vi "main 0.9.2.vi"() -> ()   [LabVIEW 2020]
uses:
  subvi/Newport ESP301/Newport ESP301.lvlib
  subvi/sp_manip.llb/sp_manip_lib.lvlib
  subvi/sp_manip.llb/tcp_gateway.lvlib
  subvi/PHOIBOS/DEFINITIONS/DEF_dev_type.ctl
  subvi/PHOIBOS/DEFINITIONS/DEF_dev_state.ctl
  <vilib>/Utility/file.llb/Write Delimited Spreadsheet (DBL).vi
  <vilib>/Utility/file.llb/Read Delimited Spreadsheet (string).vi
  <vilib>/Analysis/NI_AALBase.lvlib
  <vilib>/Analysis/1siggen.llb/Ramp Pattern by Samples.vi
  <vilib>/DAQmx/create/channels.llb/DAQmx Create Channel (AI-Voltage-Basic).vi
panel:
  in  "Frame trigger \n(High Performance and QE only)":u16
  in  "Operating mode\nHP & QE / HS & DiCam Pro":u32=1
  out "Waveform Chart":dbl(graph)=205.72
  out "G2 X":cluster{dbl[], "Ramp Pattern":dbl[]}(graph)
  in  "reset every n pics":bool=TRUE
  in  "pics2avg":i32=20
  in  "abort acq.":bool
  out "G2 Y":cluster{dbl[], "Ramp Pattern":dbl[]}(graph)={[0.0, 0.0, 0.0, 0.0, 0.0, 0.0, 0.0, 0.0, 0.0, 0.0, 0.0, 0.0, 0.0, 0.0, 0.0, 0.0, 0.0, 0.0, 0.0, 0.0, 0.0, 0.0, 0.0, 0.0, 0.0, 0.0, 0.0, 0.0, 0.0, 0.0, 0.0, 0.0, 0.0, 0.0, 0.0, 0.0, 0.0, 0.0, 0.0, 0.0, 0.0, 0.0, 0.0, 0.0, 0.0, 0.0, 0.0, 0.0, 0.0, 0.0, 0.0, 0.0, 0.0, 0.0, 0.0, 0.0, 0.0, 0.0, 0.0, 0.0, 0.0, 0.0, 0.0, 0.0, 0.0, 0.0, 0.0, 0.0, 0.0, 0.0, 0.0, 0.0, 0.0, 0.0, 0.0, 0.0, 0.0, 28.048333333333332, 101.45500000000001, 63.635000000000005, 12.581666666666669, 0.0, 0.0, 0.0, 0.0, 0.0, 0.0, 0.0, 0.0, 0.0, 0.0, 0.0, 0.0, 0.0, 0.0, 0.0, 0.0, 0.0, 0.0, 0.0, 0.0, 0.0, 0.0, 0.0, 0.0, 0.0, 0.0, 0.0, 0.0, 0.0, 0.0, 0.0, 0.0, 0.0, 0.0, 0.0, 0.0, 0.0, 0.0, 0.0, 0.0, 0.0, 0.0, 0.0, 0.0, 0.0, 0.0, 0.0, 0.0, 0.0, 0.0, 0.0, 0.0, 0.0, 0.0, 0.0, 0.0, 0.0, 0.0, 0.0, 0.0, 0.0, 0.0, 0.0, 0.0, 0.0, 0.0, 0.0, 0.0, 0.0, 0.0, 0.0, 0.0, 0.0, 0.0, 0.0, 0.0, 0.0, 0.0, 0.0, 0.0, 0.0, 0.0, 0.0, 0.0, 0.0, 0.0, 0.0, 0.0, 0.0, 0.0, 0.0, 0.0, 0.0, 0.0, 0.0, 0.0, 0.0, 0.0, 0.0, 0.0, 0.0, 0.0, 0.0, 0.0, 0.0, 0.0, 0.0, 0.0, 0.0, 0.0, 0.0, 0.0, 0.0, 0.0, 0.0, 0.0, 0.0, 0.0, 0.0, 0.0, 0.0, 0.0, 0.0, 0.0, 0.0, 0.0, 0.0, 0.0, 0.0, 0.0, 0.0, 0.0, 0.0, 0.0, 0.0, 0.0, 0.0, 0.0, 0.0, 0.0, 0.0, 0.0, 0.0, 0.0, 0.0, 0.0, 0.0, 0.0, 0.0, 0.0, 0.0, 0.0, 0.0, 0.0, 0.0, 0.0, 0.0, 0.0, 0.0, 0.0, 0.0, 0.0, 0.0, 0.0, 0.0, 0.0, 0.0, 0.0, 0.0, 0.0, 0.0, 0.0, 0.0, 0.0, 0.0], "Ramp Pattern"=[0.0, 1.003921568627451, 2.007843137254902, 3.011764705882353, 4.015686274509804, 5.019607843137255, 6.023529411764706, 7.027450980392157, 8.031372549019608, 9.035294117647059, 10.03921568627451, 11.04313725490196, 12.047058823529412, 13.050980392156863, 14.054901960784314, 15.058823529411764, 16.062745098039215, 17.066666666666666, 18.070588235294117, 19.07450980392157, 20.07843137254902, 21.08235294117647, 22.08627450980392, 23.090196078431372, 24.094117647058823, 25.098039215686274, 26.101960784313725, 27.105882352941176, 28.109803921568627, 29.113725490196078, 30.11764705882353, 31.12156862745098, 32.12549019607843, 33.129411764705885, 34.13333333333333, 35.13725490196079, 36.141176470588235, 37.14509803921569, 38.14901960784314, 39.15294117647059, 40.15686274509804, 41.16078431372549, 42.16470588235294, 43.168627450980395, 44.17254901960784, 45.1764705882353, 46.180392156862744, 47.1843137254902, 48.188235294117646, 49.1921568627451, 50.19607843137255, 51.2, 52.20392156862745, 53.207843137254905, 54.21176470588235, 55.21568627450981, 56.219607843137254, 57.22352941176471, 58.227450980392156, 59.23137254901961, 60.23529411764706, 61.23921568627451, 62.24313725490196, 63.247058823529414, 64.25098039215686, 65.25490196078431, 66.25882352941177, 67.26274509803922, 68.26666666666667, 69.27058823529411, 70.27450980392157, 71.27843137254902, 72.28235294117647, 73.28627450980392, 74.29019607843138, 75.29411764705883, 76.29803921568627, 77.30196078431372, 78.30588235294118, 79.30980392156863, 80.31372549019608, 81.31764705882352, 82.32156862745099, 83.32549019607843, 84.32941176470588, 85.33333333333333, 86.33725490196079, 87.34117647058824, 88.34509803921569, 89.34901960784313, 90.3529411764706, 91.35686274509804, 92.36078431372549, 93.36470588235294, 94.3686274509804, 95.37254901960785, 96.37647058823529, 97.38039215686274, 98.3843137254902, 99.38823529411765, 100.3921568627451, 101.39607843137254, 102.4, 103.40392156862745, 104.4078431372549, 105.41176470588235, 106.41568627450981, 107.41960784313726, 108.4235294117647, 109.42745098039215, 110.43137254901961, 111.43529411764706, 112.43921568627451, 113.44313725490196, 114.44705882352942, 115.45098039215686, 116.45490196078431, 117.45882352941176, 118.46274509803922, 119.46666666666667, 120.47058823529412, 121.47450980392156, 122.47843137254903, 123.48235294117647, 124.48627450980392, 125.49019607843137, 126.49411764705883, 127.49803921568628, 128.50196078431372, 129.50588235294117, 130.50980392156862, 131.51372549019607, 132.51764705882354, 133.521568627451, 134.52549019607844, 135.52941176470588, 136.53333333333333, 137.53725490196078, 138.54117647058823, 139.54509803921567, 140.54901960784315, 141.5529411764706, 142.55686274509804, 143.5607843137255, 144.56470588235294, 145.5686274509804, 146.57254901960783, 147.57647058823528, 148.58039215686276, 149.5843137254902, 150.58823529411765, 151.5921568627451, 152.59607843137255, 153.6, 154.60392156862744, 155.6078431372549, 156.61176470588236, 157.6156862745098, 158.61960784313726, 159.6235294117647, 160.62745098039215, 161.6313725490196, 162.63529411764705, 163.6392156862745, 164.64313725490197, 165.64705882352942, 166.65098039215687, 167.65490196078431, 168.65882352941176, 169.6627450980392, 170.66666666666666, 171.6705882352941, 172.67450980392158, 173.67843137254903, 174.68235294117648, 175.68627450980392, 176.69019607843137, 177.69411764705882, 178.69803921568626, 179.7019607843137, 180.7058823529412, 181.70980392156864, 182.71372549019608, 183.71764705882353, 184.72156862745098, 185.72549019607843, 186.72941176470587, 187.73333333333332, 188.7372549019608, 189.74117647058824, 190.7450980392157, 191.74901960784314, 192.75294117647059, 193.75686274509803, 194.76078431372548, 195.76470588235293, 196.7686274509804, 197.77254901960785, 198.7764705882353, 199.78039215686275, 200.7843137254902, 201.78823529411764, 202.7921568627451, 203.79607843137254, 204.8, 205.80392156862746, 206.8078431372549, 207.81176470588235, 208.8156862745098, 209.81960784313725, 210.8235294117647, 211.82745098039214, 212.83137254901962, 213.83529411764707, 214.8392156862745, 215.84313725490196, 216.8470588235294, 217.85098039215686, 218.8549019607843, 219.85882352941175, 220.86274509803923, 221.86666666666667, 222.87058823529412, 223.87450980392157, 224.87843137254902, 225.88235294117646, 226.8862745098039, 227.89019607843136, 228.89411764705883, 229.89803921568628, 230.90196078431373, 231.90588235294118, 232.90980392156862, 233.91372549019607, 234.91764705882352, 235.92156862745097, 236.92549019607844, 237.9294117647059, 238.93333333333334, 239.93725490196078, 240.94117647058823, 241.94509803921568, 242.94901960784313, 243.95294117647057, 244.95686274509805, 245.9607843137255, 246.96470588235294, 247.9686274509804, 248.97254901960784, 249.9764705882353, 250.98039215686273, 251.98431372549018, 252.98823529411766, 253.9921568627451, 254.99607843137255, 256.0]}
  out "ETA":timestamp=timestamp(3548431207.455768 s since 1904-01-01) format="%<%H:%M:%S>T"
  out "acq. imgs":i32=50
  out "snap_prog":dbl(slide)=1.0 scale=0.0..1.0
  in  "BasePath":path=path "Z:/PESdata"
  in  "cam_liveavg":bool=TRUE caption="live average"
  out "cam_fps":dbl=19.76375300099574 caption="FPS" format="%.1g"
  out "sideimg":dbl[][](graph)
  in  "RunNumber":u16=145
  out "sum":dbl=205.72 format="%#.2g"
  out "max":dbl=120.33666666666666
  out "mainimg":dbl[][](graph)
  out "ESP_con?":bool=TRUE caption="ESP301"
  out "phoib_con?":bool caption="PHOIBOS"
  out "manip_con?":bool caption="manipulator"
  out "cam_con?":bool caption="camera"
  in  "main_close":bool
  in  "Tab Control":T1(tab)
  in  "manip_deltas":dbl[](array[numeric])=[0.0, 0.0, 0.0, 0.0, 10.0, 0.0] caption="delta" format="%#.5g"
  in  "aq.mode":enum32{"Radio Selection 1", "Radio Selection 2"}(radio)=enum."Radio Selection 2"
  in  "dark avg":i32=100
  in  "averages":i32=50 caption="N"
  in  "ESP_delta":dbl=0.0015 caption="relative [mm]"
  in  "ESP_-":bool
  in  "ESP_+":bool
  in  "ESP_go":bool
  in  "ESP_dest_t":dbl=-1000.0 caption="[fs]"
  in  "ESP_dest":dbl=26.730803771 caption="[mm]"
  in  "ESP_set_t0":bool
  in  "phoib_I_6s":dbl=3200.0
  in  "phoib_I_5s":dbl=1500.0
  in  "phoib_I_4s":dbl=4.558
  in  "phoib_I_3s":dbl=-7.0
  in  "phoib_I_2s":dbl=20.0
  in  "phoib_I_1s":dbl=22.0
  in  "phoib_standby":bool
  in  "phoib_set":bool
  out "phoib_I_6":dbl=3200.0 caption="Screen Voltage"
  out "phoib_I_5":dbl=1500.0 caption="Detctor Voltage"
  out "phoib_I_4":dbl=4.558 caption="Work Function"
  out "phoib_I_3":dbl=-7.0 caption="Coil Current"
  out "phoib_I_2":dbl=20.0 caption="Pass Energy"
  out "phoib_I_1":dbl=22.0 caption="Kinetic Energy"
  out "Saved Positions":string[][](table)=[["ertwertwert", "-2.299945", "-2.030214", "38.900024", "50.000762", "0.000887", "-97.998082"], ["uztgugt", "-14.999451", "-13.638894", "442.380066", "13.998380", "-1.893758", "-76.305838"], ["asdf", "-14.999451", "-13.638894", "442.380066", "13.998380", "-1.893758", "-76.305838"], ["test3", "-14.999451", "-13.638894", "441.380066", "13.998380", "-1.893758", "-76.305838"]]
  in  "Save Pos":bool
  in  "Load":bool
  in  "Delete":bool
  in  "ManipRel +":bool
  in  "ManipRel -":bool
  in  "Move Abs":bool
  in  "stop manip":bool
  in  "dest":dbl[](array[numeric])=[-2.6172862113166087, -0.009888298846365134, 68.5008544921875, -46.36280498847848, 1.1073518432055398, -218.56360350415366] caption="destination" format="%#.5g"
  out "axis":string[](array[string])=["x", "y", "z", "polar", "tilt", "azimut"]
  out "pos":dbl[](array[numeric]) caption="position" format="%.5f"
  in  "Mode":T2(ring)=enum."WideAngleMode"
  in  "VoltageRange":enum16{"3.5kV", "1.5kV", "400V", "100V", "10V"}(ring)=enum."400V"
  out "ESP_pos":dbl=26.86195 caption="Position"
  out "ESP_delay":dbl=-125.08653569931175 caption="Delay"
  out "ESP_t0":dbl=26.8807 caption="Time Zero @"
  out "phoib_I_7":dbl=-17.0 caption="Conversion Voltage"
  in  "phoib_I_7s":dbl=-17.0
  in  "phoib_I_8s":dbl=0.0039
  in  "phoib_I_9s":dbl=0.0039
  out "phoib_I_8":dbl=0.0039 caption="FD1"
  out "phoib_I_9":dbl=0.0039 caption="FD2"
  in  "gain":bool
  in  "exposure [ms]":u32=50
  in  "binning":u16(ring)=2 items=["X 1", "X 2", "X 4", "X 8"]
  in  "cam_dark?":bool=TRUE caption="subtract dark?"
  in  "cam_dark":bool
  in  "cam_saveimg":bool
  in  "e-size":u8
  in  "lower threshold":i32=50
  in  "count?":bool
  in  "ROI Left":i32=1
  in  "ROI Right":i32=43
  in  "ROI Top":i32=1
  in  "ROI Bottom":i32=33
  out "moving?":bool[](array[boolean])
  out "del_ETA":timestamp=timestamp(3548447168.6093655 s since 1904-01-01) format="%<%H:%M:%S>T"
  out "time / step":dbl=3.7475930503989816
  out "duration [HH:MM:SS]":dbl=47385.71071624756 format="%<%H:%M:%S>t"
  out "disk [MB]":dbl=5419.953
  out "RAM [MB]":dbl=27.097
  out "total steps":dbl=9800.0
  out "delaypoints":dbl=49.0
  in  "generate delay table":bool
  in  "load delay table":bool
  in  "delay table [fs]":string[][](table)=[["-200.000000"], ["-175.000000"], ["-150.000000"], ["-125.000000"], ["-100.000000"], ["-75.000000"], ["-50.000000"], ["-25.000000"], ["0.000000"], ["25.000000"], ["50.000000"], ["75.000000"], ["100.000000"], ["125.000000"], ["150.000000"], ["175.000000"], ["200.000000"], ["225.000000"], ["250.000000"], ["275.000000"], ["300.000000"], ["325.000000"], ["350.000000"], ["375.000000"], ["400.000000"], ["425.000000"], ["450.000000"], ["475.000000"], ["500.000000"], ["525.000000"], ["550.000000"], ["575.000000"], ["600.000000"], ["625.000000"], ["650.000000"], ["675.000000"], ["700.000000"], ["725.000000"], ["750.000000"], ["775.000000"], ["800.000000"], ["825.000000"], ["850.000000"], ["875.000000"], ["900.000000"], ["925.000000"], ["950.000000"], ["975.000000"], ["1000.000000"]]
  in  "delscan_iters":u32=200 caption="iterations"
  out "scangraph":cluster{"delaypoints":dbl[], dbl[]}(graph)={"delaypoints"=[-200.0, -175.0, -150.0, -125.0, -100.0, -75.0, -50.0, -25.0, 0.0, 25.0, 50.0, 75.0, 100.0, 125.0, 150.0, 175.0, 200.0, 225.0, 250.0, 275.0, 300.0, 325.0, 350.0, 375.0, 400.0, 425.0, 450.0, 475.0, 500.0, 525.0, 550.0, 575.0, 600.0, 625.0, 650.0, 675.0, 700.0, 725.0, 750.0, 775.0, 800.0, 825.0, 850.0, 875.0, 900.0, 925.0, 950.0, 975.0, 1000.0], [21425.231929824553, 20846.290614035148, 20035.560438596513, 18931.235614035082, 19640.659557522133, 21305.676814159116, 29251.80778761067, 69089.9434513275, 126421.4030973446, 163646.65610619384, 171927.22929203612, 157521.9204424778, 146716.11486725596, 135894.3418584061, 130437.91398230121, 119156.57761061934, 115502.62300884936, 103421.47973451365, 100060.49123893768, 93085.71787610617, 90135.85805309749, 86817.93584070833, 80391.69256637139, 77159.11646017693, 77729.56053097341, 73257.13840707966, 70575.97486725691, 66315.25460177004, 66705.37823008854, 63696.19292035409, 61819.46247787618, 60200.33123893791, 57469.7140707966, 55306.85336283208, 53731.13327433622, 50220.71699115046, 51078.037433628335, 47817.420265486544, 47812.83389380534, 46146.23106194685, 44534.275398229904, 42332.0369026551, 45537.85681415925, 40834.3, 41967.50035398256, 40596.04380530956, 39278.89221238937, 39217.73823008859, 37653.17115044236]}
  in  "delscan_abort":bool
  out "delscan_progress":u32(slide)=4 scale=0.0..49.0
  in  "delscan_go":bool
  out "delscan_pos":dbl=26.861962971375 caption="stage pos [mm]"
  in  "delscan_end":dbl=1000.0 caption="end [fs]"
  in  "delscan_stepsize":dbl=25.0 caption="stepsize [fs]"
  in  "delscan_start":dbl=-200.0 caption="start [fs]"
  out "iteration":i32=114
  in  "delscan_finishIteration":bool
  in  "manip_scan_steps":u32=3
  in  "Optimize":bool
  in  "manip_scan_delta":dbl[](array[numeric])=[0.0, 0.0, 0.0, 0.0, 1.0, 0.0] caption="delta" format="%#.5g"
  out "delscan_progress 2":u32(slide)=2 scale=0.0..3.0
  in  "abort":bool
  in  "dev_bench":bool
  out "x/y":dbl
  out "1/x":dbl
  in  "stop":bool
  out "voltage out":dbl
  out "sideimg 2":i32[][](graph)
  in  "manip_init":bool
  in  "manip_release":bool
  in  "phoib_init":bool
  in  "phoib_release":bool
  in  "ESP_init":bool
  in  "ESP_release":bool
  in  "ESP301 VISA":refnum<visa-resource-name>="COM8"
  in  "board number":i32
  in  "cam_init":bool
  in  "cam_release":bool
  out "cam_error":errorcluster
  out "phoib_error":errorcluster
  out "state":T3=1 items=["Off"=-1, "Standby"=0, "On"=1]
  in  "ESP Axis":i32=1 min=1 max=3
  out "error out":errorcluster
  out "error out 2":errorcluster={"status"=TRUE, "code"=1, "source"="TCP Write in sp_manip_lib.lvlib:sp_manip_disconnect.vi->main 0.9.2.vi"}
  # "0 = sequential\n1 = simultaneous"
  # "0 = internal\n1 = external rising\n2 = external falling"
  # "camera"
  # "analyzer"
  # "manipulator"
  # "aquisition"
  # "delay stage"
  # "Position"
  # "Destination"
  # "X\nY\nZ\npolar\ntilt\nazimut"
  # "camera"
  # "phoibos"
  # "ESP301"
  # "manipulator"
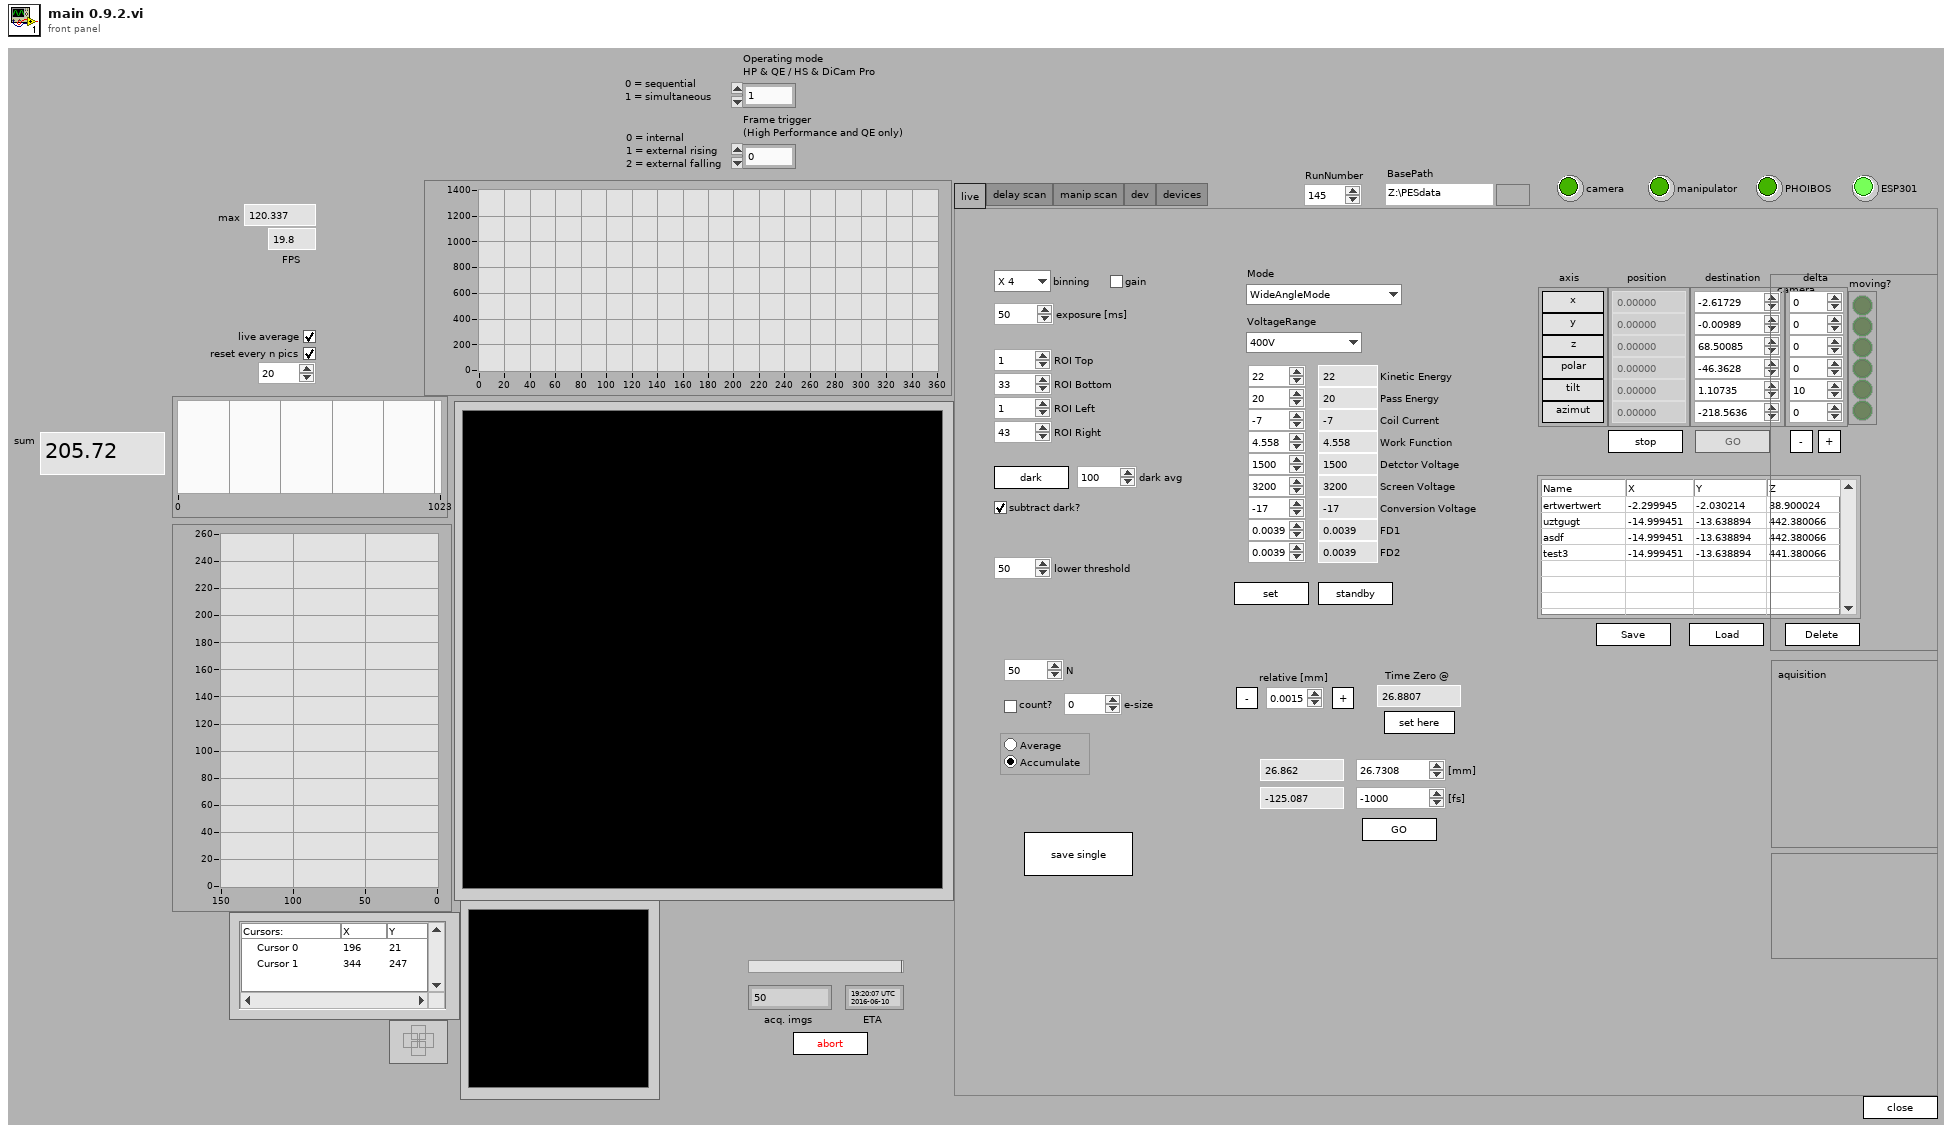
[diagram p1: front panel]
types:
  T1 = enum32{"live", "delay scan", "manip scan", "dev", "devices"}
  T2 = enum16{"HighMagnification", "MediumMagnification", "LowMagnification", "HighAngularDispersion", "MediumAngularDispersion", "LowAngularDispersion", "WideAngleMode", "LargeArea", "MediumArea", "SmallArea", "HighMagnification2", "SmallArea2", "ImagingMode"}
  T3 = typedef "DEF_dev_state.ctl" = i32
  T4 = typedef "LVCursorListTypeDef.ctl" = cluster{"Name":string, "Color":u32, "Style":u8, "Point Style":u8, "Name Visible":bool, "Allow Drag":bool, "Cursor Mode":u32, "Plot":i32, "Index":i32, "Position":cluster{"X":dbl, "Y":dbl}, "X Scale":u32, "Y Scale":u32, "Watch Plots":i32[], "Watch All Plots":bool, "Plot Area":i32, "Label Offset":cluster{"X":dbl, "Y":dbl}}[]
  T5 = cluster{"delay pointss [fs]":dbl[], "Intensity Chart":dbl[]}
  T6 = cluster{"Camera type":u32, "Operating mode\nHP & QE / HS & DiCam Pro ":u32, "Frame trigger \n(High Performance and QE only)":u16, "Sequence trigger":u16, "Low Light\n(QE only)":bool, "Gain":bool, "Horzontal\nbinning":u16, "Vertical\nbinning ":u16, "ROI Left":i32, "ROI Right":i32, "ROI Top":i32, "ROI Bottom":i32}
  T7 = cluster{"Name":string, "Color":u32, "Style":u8, "Point Style":u8, "Name Visible":bool, "Allow Drag":bool, "Cursor Mode":u32, "Plot":i32, "Index":i32, "Position":cluster{"X":dbl, "Y":dbl}, "X Scale":u32, "Y Scale":u32, "Watch Plots":i32[], "Watch All Plots":bool, "Plot Area":i32, "Label Offset":cluster{"X":dbl, "Y":dbl}}
  T8 = cluster{"Axis_Name":string, "Axis_Type":string, "Axis_Position":dbl, "continous":bool, "moving":bool}[]
  T9 = typedef "DEF_dev_type.ctl" = enum32{"devA (analyzer)", "devD (detector)"}
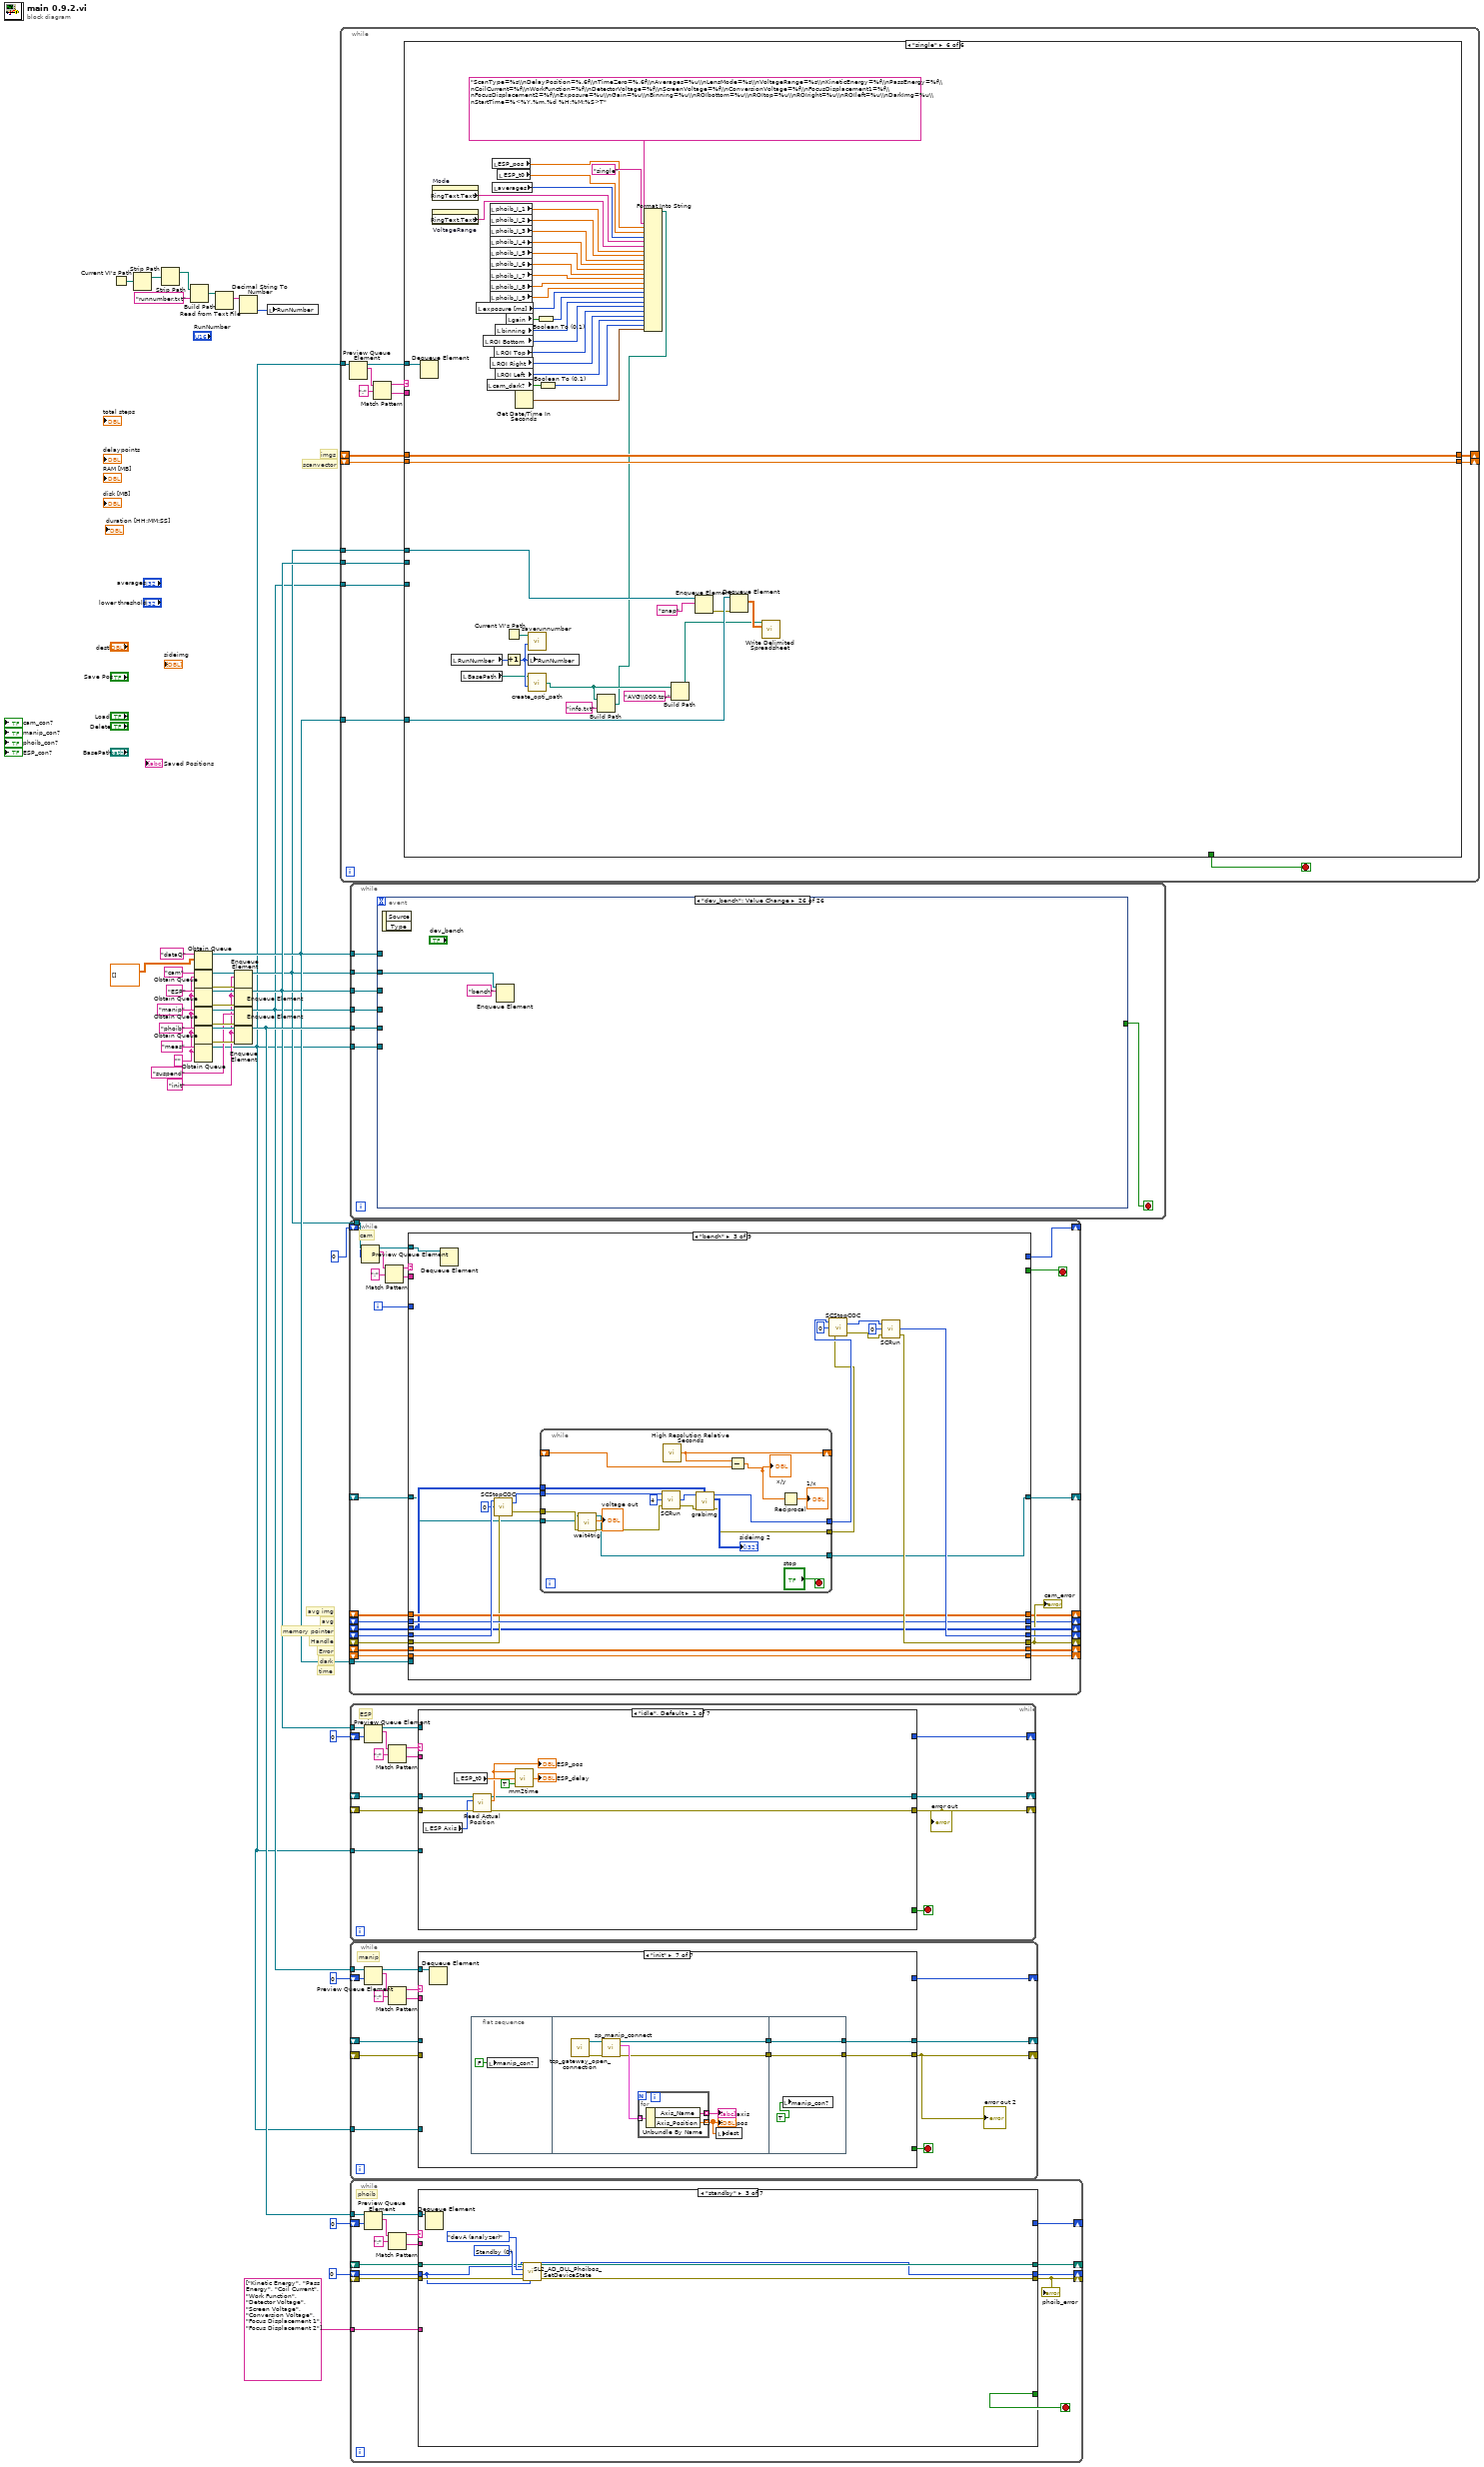
[diagram p0: block diagram]
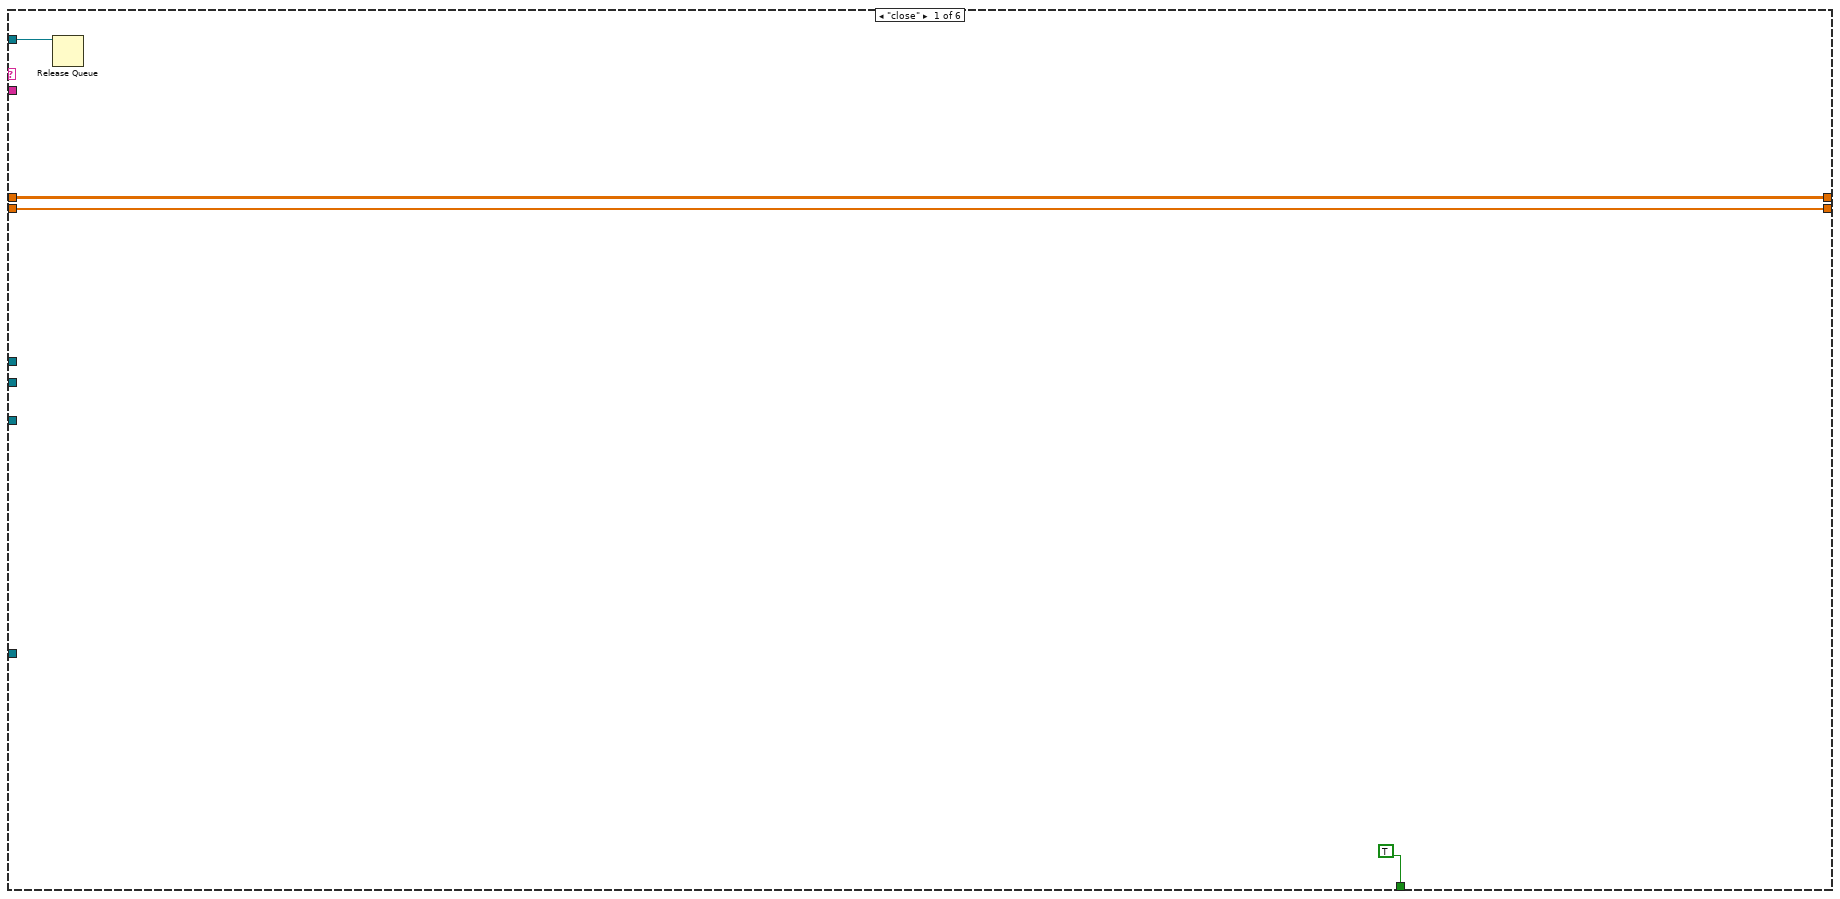
[diagram p2: hidden frame]
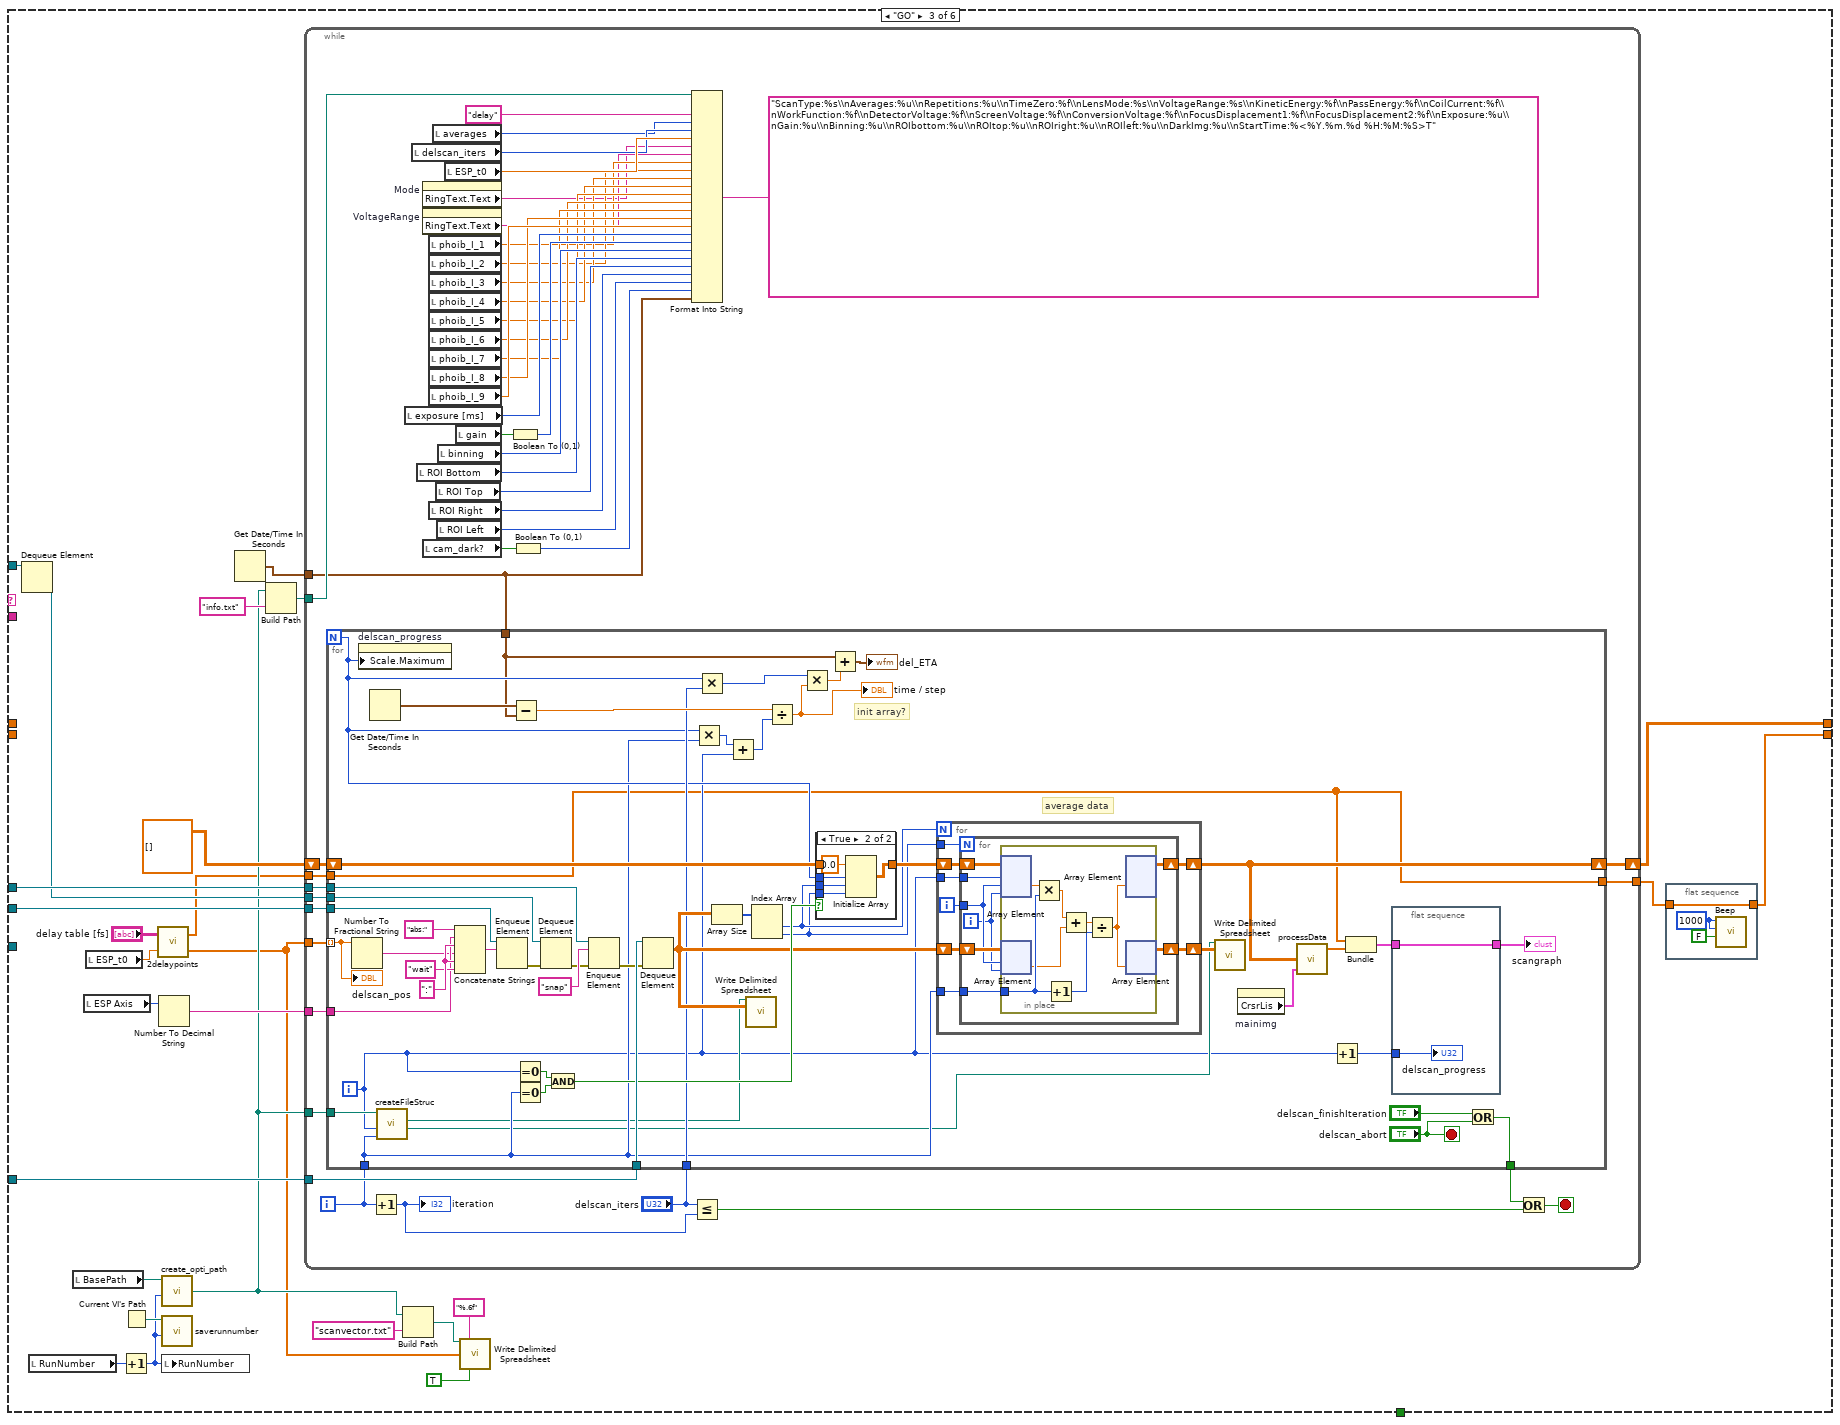
[diagram p4: hidden frame]
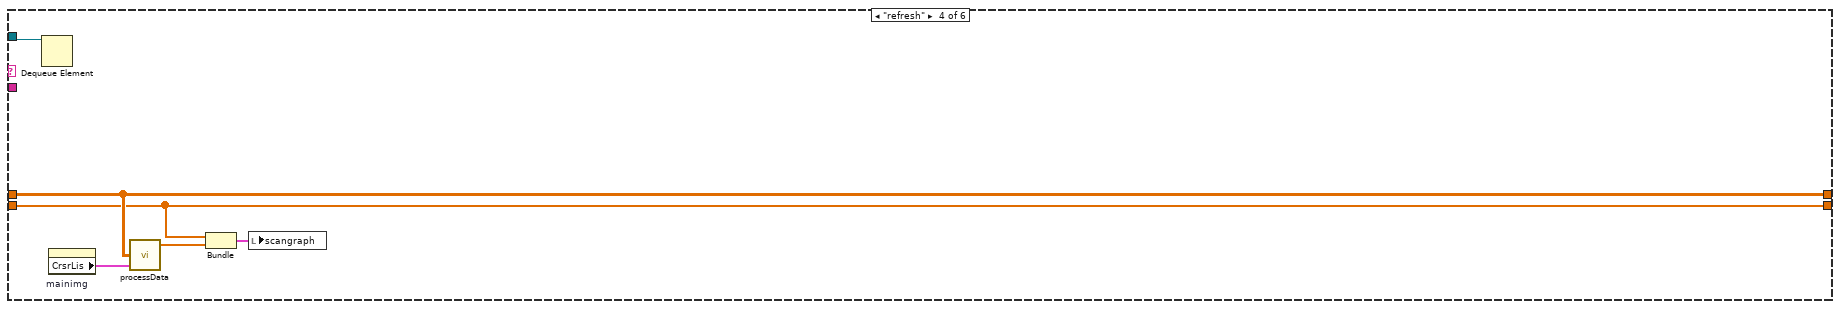
[diagram p6: hidden frame]
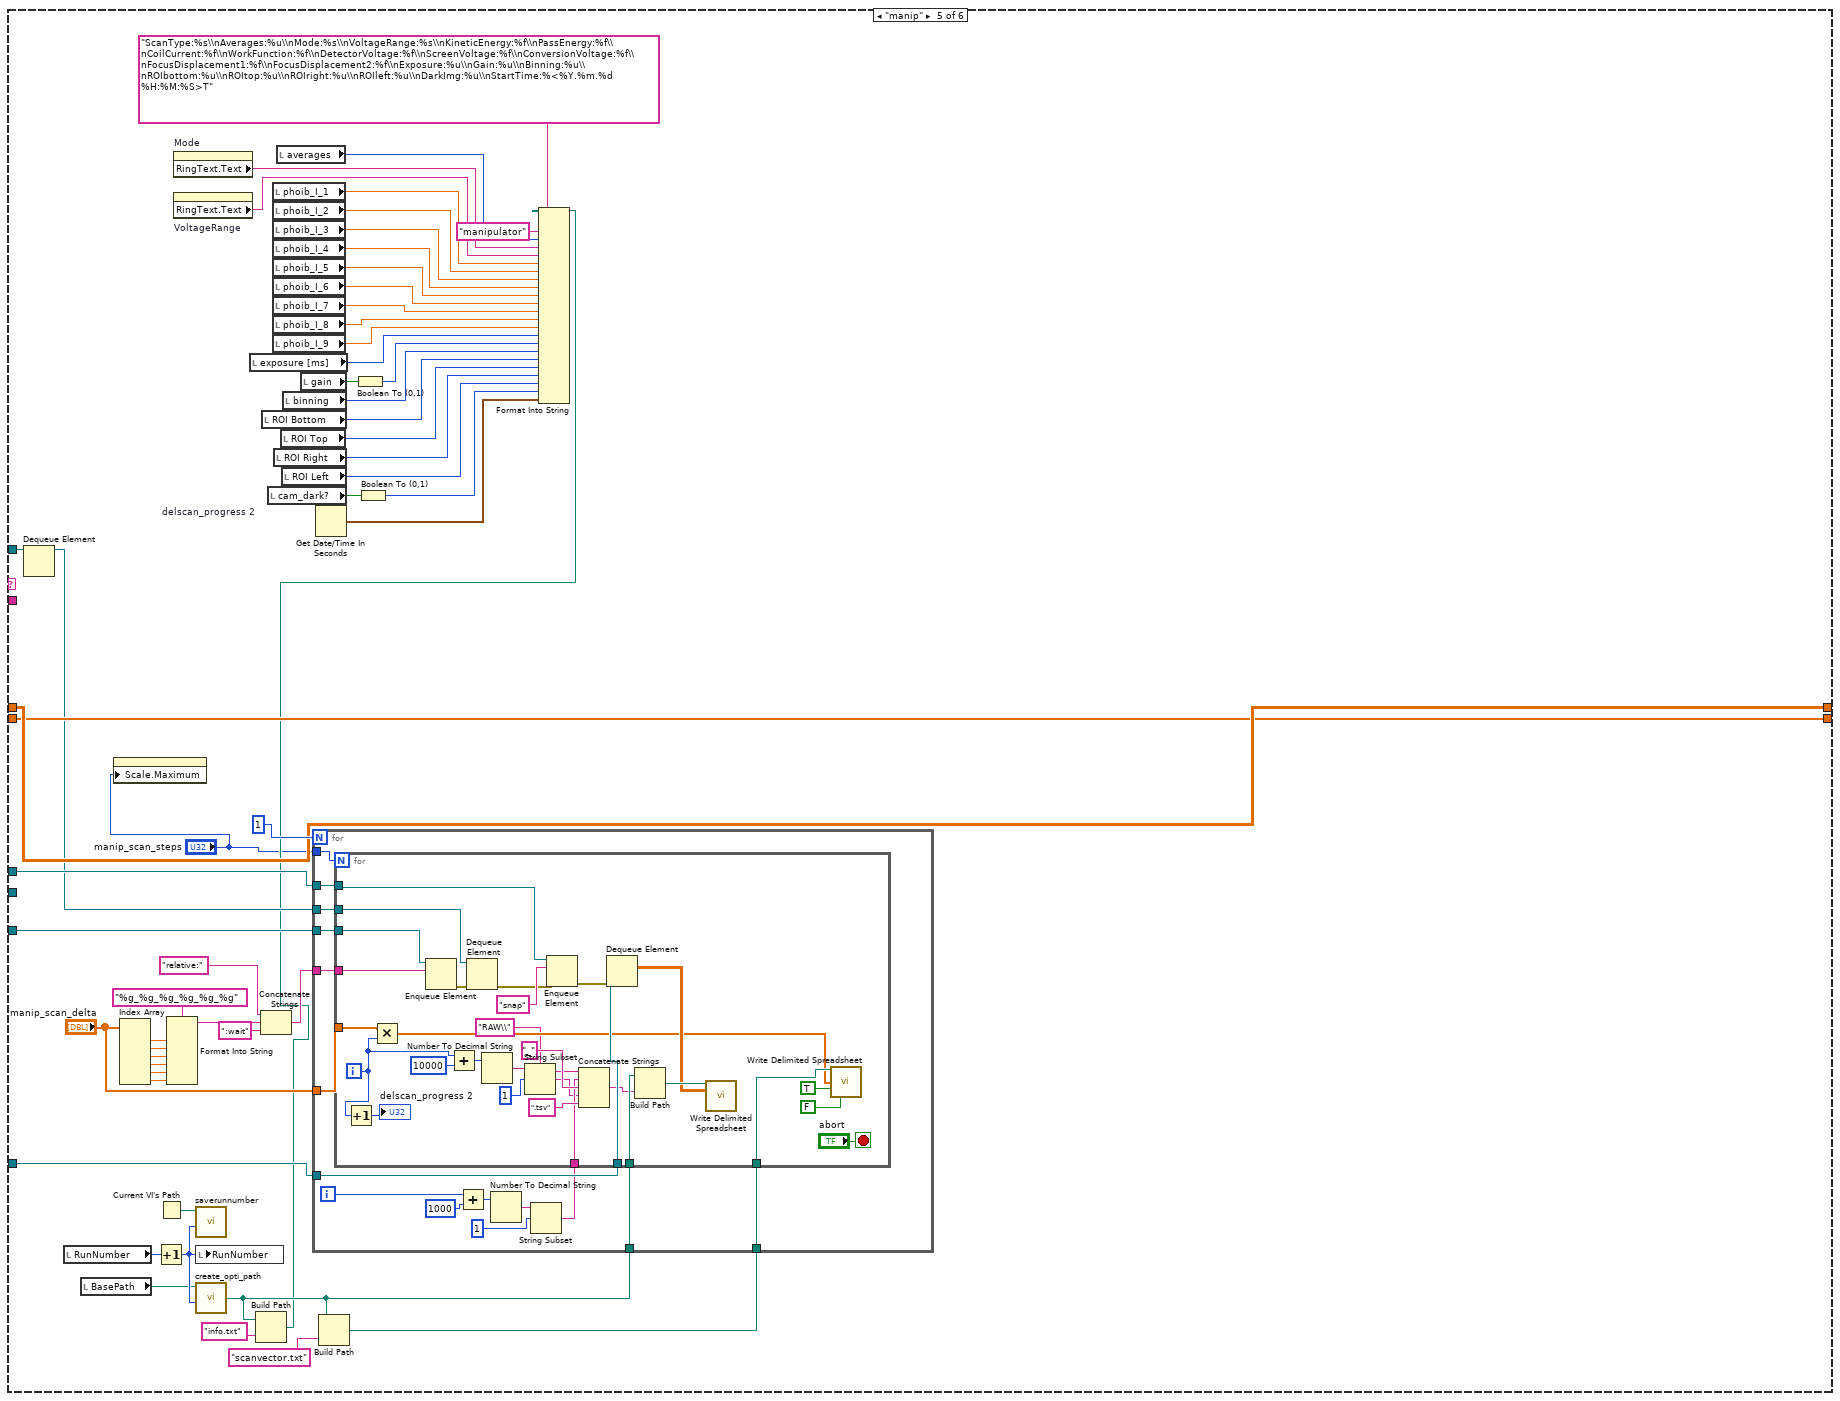
[diagram p7: hidden frame]
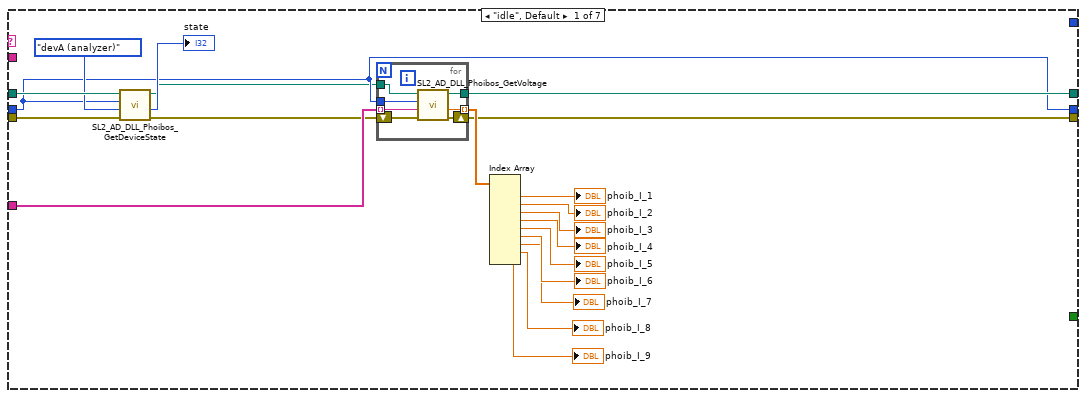
[diagram p8: hidden frame]
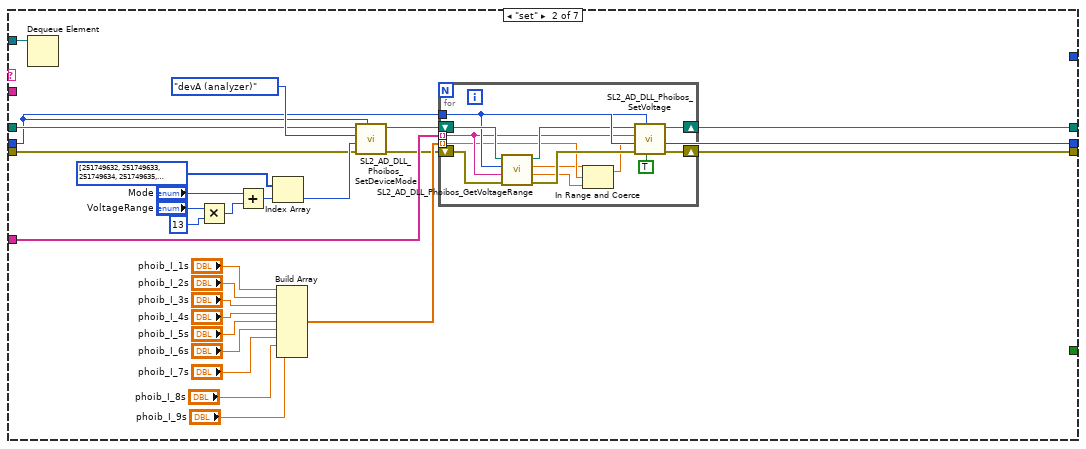
[diagram p9: hidden frame]
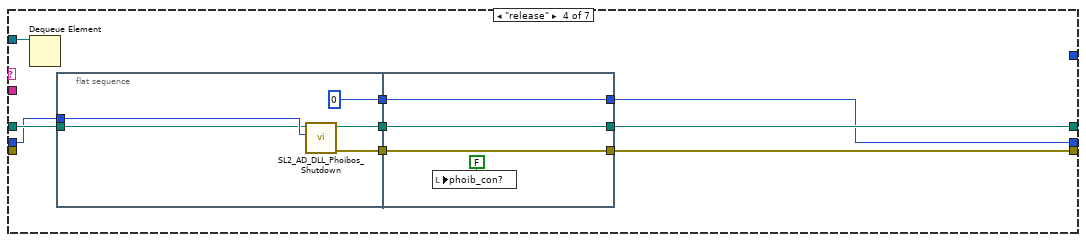
[diagram p10: hidden frame]
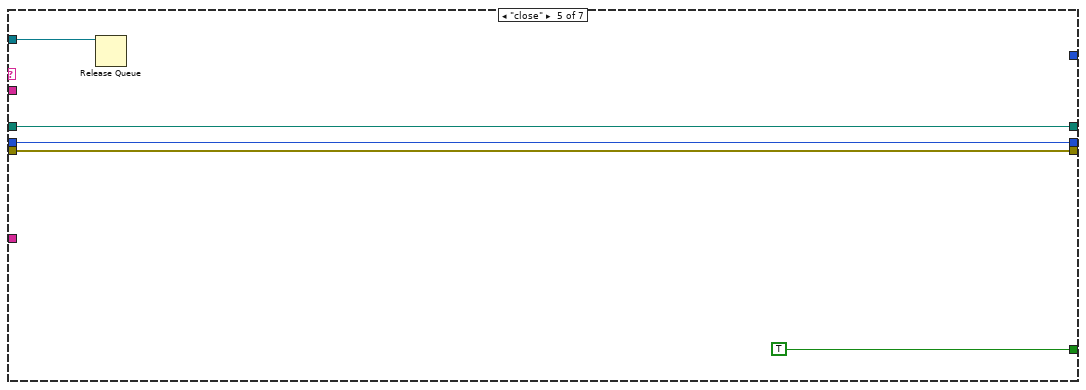
[diagram p11: hidden frame]
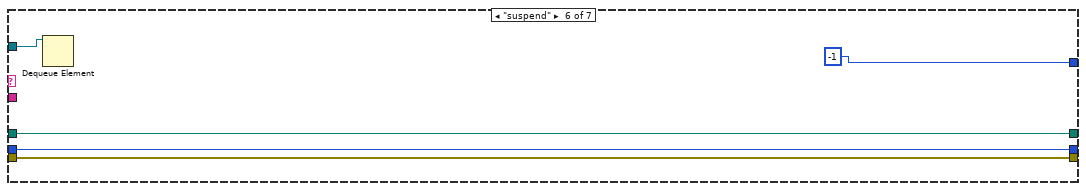
[diagram p12: hidden frame]
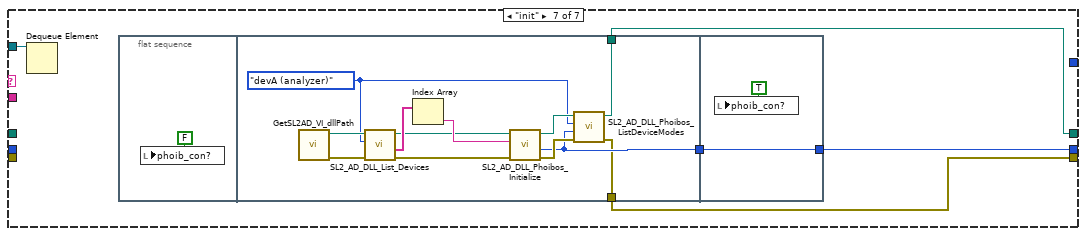
[diagram p13: hidden frame]
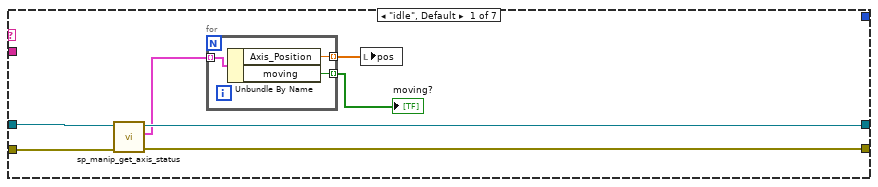
[diagram p14: hidden frame]
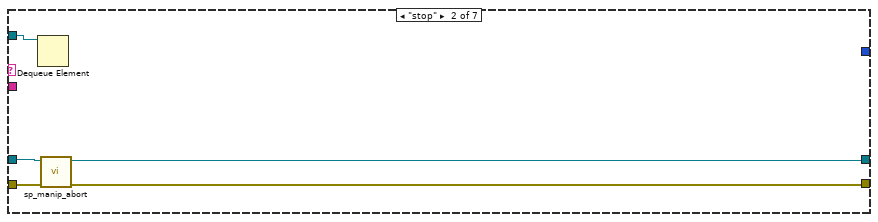
[diagram p15: hidden frame]
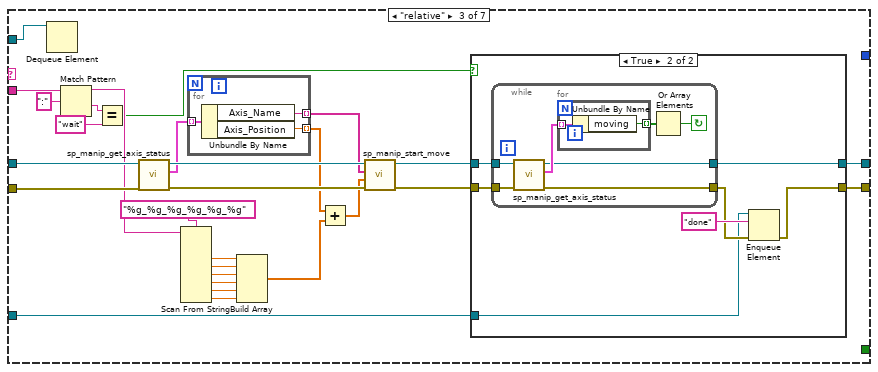
[diagram p16: hidden frame]
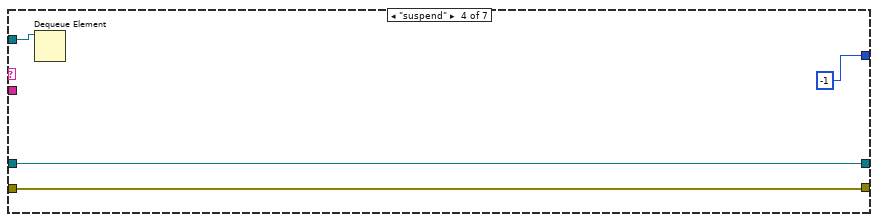
[diagram p18: hidden frame]
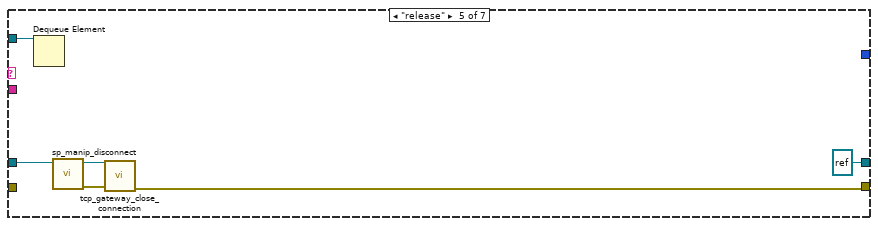
[diagram p19: hidden frame]
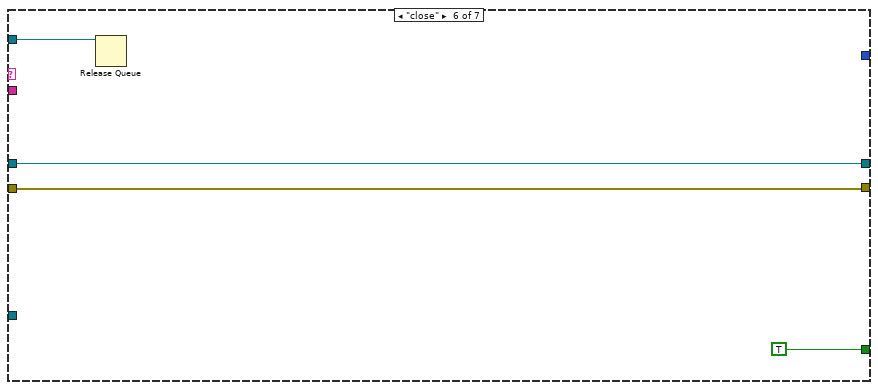
[diagram p20: hidden frame]
diagram:
  w14 = "init" ("name (unnamed)")
  w16 = "" ("name (unnamed)")
  # "scanvector"
  # "imgs"
  # "avg img"
  # "avg"
  # "time"
  # "dark"
  # "Error"
  # "Handle"
  # "memory pointer"
  n1 = Current VI's Path() -> (path=w4:path)
  n2 = Strip Path(path=w4) -> (stripped path=w8:path)  [unwired: 1 out]
  n3 = Strip Path(path=w8) -> (stripped path=w9:path)  [unwired: 1 out]
  n4 = Build Path(base path=w9, name or relative path="runnumber.txt") -> (appended path=w6:path)
  n5 = Obtain Queue(name (unnamed)="dataQ", element data type=dbl[][] []) -> (queue out=w11:refnum<queue>)  [unwired: 3 in, 2 out]
  n6 = Obtain Queue(name (unnamed)="cam", element data type=w16) -> (queue out=w36:refnum<queue>, error out=w35:errorcluster)  [unwired: 3 in, 1 out]
  n7 = Obtain Queue(name (unnamed)="ESP", element data type=w16) -> (queue out=w33:refnum<queue>, error out=w34:errorcluster)  [unwired: 3 in, 1 out]
  n8 = Obtain Queue(name (unnamed)="manip", element data type=w16) -> (queue out=w30:refnum<queue>, error out=w29:errorcluster)  [unwired: 3 in, 1 out]
  n9 = Obtain Queue(name (unnamed)="phoib", element data type=w16) -> (queue out=w27:refnum<queue>, error out=w28:errorcluster)  [unwired: 3 in, 1 out]
  n10 = Obtain Queue(name (unnamed)="meas", element data type=w16) -> (queue out=w2:refnum<queue>)  [unwired: 3 in, 2 out]
  n11 = Read from Text File(file (use dialog)=w6) -> (text=w7:string)  [unwired: 3 in, 3 out]
  n12 = Enqueue Element(queue=w36, element=w14, error in (no error)=w35) -> (queue out=w10:refnum<queue>)  [unwired: 1 in, 2 out]
  n13 = Enqueue Element(queue=w33, element=w14, error in (no error)=w34) -> (queue out=w13:refnum<queue>)  [unwired: 1 in, 2 out]
  n14 = Enqueue Element(queue=w30, element="suspend" ("name (unnamed)"), error in (no error)=w29) -> (queue out=w3:refnum<queue>)  [unwired: 1 in, 2 out]
  n15 = Enqueue Element(queue=w27, element=w14, error in (no error)=w28) -> (queue out=w24:refnum<queue>)  [unwired: 1 in, 2 out]
  n16 = Decimal String To Number(string=w7) -> (number=w1:i32)  [unwired: 2 in, 1 out]
  n17 = local write "RunNumber"(w1) -> ()
  n18 = while {
    tunnel: w11 -> [w52]
    tunnel: w13 -> [w51]
    tunnel: w10 -> [w50]
    shift-right: [w47] -> _
    shift-left: _ -> [w49]
    shift-right: [w46] -> _
    shift-left: _ -> [w48]
    tunnel: w2 -> [w43]
    tunnel: w3 -> [w38]
    stop <- w39 stop-if-true
    n19 = Preview Queue Element(queue=w43) -> (queue out=w40:refnum<queue>, element=w45:string)  [unwired: 2 in, 2 out]
    n20 = Match Pattern(string=w45, regular expression=":") -> (before substring=w42:string, after substring=w41:string)  [unwired: 1 in, 2 out]
    n21 = case shown="\"single\"" w42 {
      tunnel: w52 -> [_ _ w85 _ w258 w363]
      tunnel: w51 -> [_ _ w84 _ _ _]
      tunnel: w50 -> [_ _ w83 _ w257 w365]
      tunnel: w49 -> [w54 w58 _ w219 w254 w362]
      tunnel: w48 -> [w53 w57 _ w217 w253 w361]
      tunnel: [w54 w58 w82 w219 w254 w362] -> w47
      tunnel: [w53 w57 w65 w217 w253 w361] -> w46
      tunnel: w41 -> [_ _ _ _ _ _]
      tunnel: w40 -> [w56 _ w74 w221 w252 w364]
      tunnel: [TRUE _ _ _ _ _] -> w39
      tunnel: w38 -> [_ _ _ _ w256 _]
      frame "close" {
        n22 = Release Queue(queue=w56) -> ()  [unwired: 2 in, 3 out]
      }
      frame "idle", Default {
      }
      frame "GO" {
        n23 = Dequeue Element(queue=w74) -> (queue out=w73:refnum<queue>)  [unwired: 2 in, 3 out]
        n24 = local read "RunNumber"() -> (w80:u16)
        n25 = local read "BasePath"() -> (w79:path)
        n26 = local read "ESP Axis"() -> (w77:i32)
        n27 = local read "ESP_t0"() -> (w63:dbl)
        n28 = Increment(x=w80) -> (x+1=w78:u16)
        n29 = Current VI's Path() -> (path=w81:path)
        n30 = call "2delaypoints.vi"("Offset (mm)"=w63, "delay table [fs]"="delay table [fs]") -> ("delay points [mm]"=w62:dbl[], "delay pointss [fs]"=w60:dbl[])
        n31 = Number To Decimal String(number=w77) -> (decimal integer string=w76:string)  [unwired: 1 in]
        n32 = call "create_opti_path.vi"("RunNumber"=w78, "base path"=w79) -> ("Path"=w70:path)  [unwired: 2 in]
        n33 = call "saverunnumber.vi"("RunNumber"=w78, "VI path"=w81) -> ()  [unwired: 10 in]
        n34 = local write "RunNumber"(w78) -> ()
        n35 = Get Date/Time In Seconds() -> (seconds since 1Jan1904=w59:timestamp)
        n36 = Build Path(base path=w70, name or relative path="info.txt") -> (appended path=w61:path)
        n37 = while {
          tunnel: w62 -> [w122]
          tunnel: w76 -> [w130]
          tunnel: w84 -> [w129]
          tunnel: w85 -> [w128]
          tunnel: w73 -> [w127]
          tunnel: w83 -> [w126]
          tunnel: w70 -> [w125]
          shift-right: [w123] -> w82
          shift-left: dbl[][][] [] -> [w124]
          tunnel: [w121] -> w66
          tunnel: w61 -> [w88]
          tunnel: w60 -> [w87]
          tunnel: w59 -> [w86]
          i -> [w120]
          stop <- w116 stop-if-true
          n38 = for {
            N -> [w150]
            tunnel: w122 -> [w159] mode=indexing
            tunnel: w130 -> [w176]
            tunnel: w129 -> [w175]
            tunnel: w128 -> [w170]
            tunnel: w127 -> [w174]
            tunnel: w126 -> [w173]
            tunnel: w125 -> [w144]
            shift-right: [w134] -> w123
            shift-left: w124 -> [w166]
            tunnel: w120 -> [w143]
            tunnel: w87 -> [w132]
            tunnel: [w132] -> w121
            tunnel: [w156] -> w118
            tunnel: w86 -> [w146]
            tunnel: "delscan_iters" -> [w151]
            i -> [w136]
            stop <- "delscan_abort" stop-if-true
            w178 = ":" ("string")
            # "average data"
            # "init array?"
            n39 = Number To Fractional String(number=w159) -> (F-format string=w168:string)  [unwired: 3 in]
            n40 = property on="delscan_progress" class="Slide (strict)"("Scale.Maximum"=w150) -> ()  [unwired: 2 in, 2 out]
            n41 = Get Date/Time In Seconds() -> (seconds since 1Jan1904=w154:timestamp)
            n42 = call "createFileStruc.vi"("i_iter"=w143, "i_delay"=w136, "meas_path"=w144) -> ("AVG file"=w139:path, "RAW file"=w140:path)  [unwired: 7 in]
            n43 = Concatenate Strings("abs:" ("string"), w176, w178, w168, w178, "wait" ("string")) -> (w181:string)
            n44 = Enqueue Element(queue=w175, element=w181) -> (error out=w179:errorcluster)  [unwired: 2 in, 2 out]
            n45 = Subtract(x=w154, y=w146) -> (x-y=w152:dbl)
            n46 = Equal To 0?(x=w136) -> (x = 0?=w142:bool)
            n47 = Equal To 0?(x=w143) -> (x = 0?=w141:bool)
            n48 = Dequeue Element(queue=w174, error in (no error)=w179) -> (error out=w171:errorcluster)  [unwired: 1 in, 3 out]
            n49 = And(x=w142, y=w141) -> (x .and. y?=w167:bool)
            n50 = Enqueue Element(queue=w173, element="snap", error in (no error)=w171) -> (error out=w169:errorcluster)  [unwired: 1 in, 2 out]
            n51 = Dequeue Element(queue=w170, error in (no error)=w169) -> (element=w162:dbl[][])  [unwired: 1 in, 3 out]
            n52 = Multiply(x=w150, y=w143) -> (x*y=w155:i32)
            n53 = Multiply(x=w150, y=w151) -> (x*y=w149:u32)
            n54 = Array Size(array=w162) -> (size(s)=w163:i32[])
            n55 = Add(x=w155, y=w136) -> (x+y=w153:i32)
            n56 = call-poly <vilib>:"Write Delimited Spreadsheet.vi"("file path (dialog if empty)"=w140, "2D data"=w162) -> ()  [unwired: 12 in, 2 out]
            n57 = Index Array(array=w163) -> (element #1=w161:i32, element #2=w160:i32)  [unwired: 2 in]
            n58 = Divide(x=w152, y=w153) -> (x/y=w148:dbl)
            "time / step" <- w148
            n59 = Multiply(x=w149, y=w148) -> (x*y=w147:dbl)
            n60 = case shown="True" w167 {
              tunnel: w150 -> [_ w189]
              tunnel: [w184 w187] -> w165
              tunnel: w166 -> [w184 _]
              tunnel: w161 -> [_ w186]
              tunnel: w160 -> [_ w185]
              frame False {
              }
              frame True {
                n61 = Initialize Array(0.0 ("element"), w189, w186, w185) -> (w187:dbl[][][])
              }
            }
            n62 = Add(x=w146, y=w147) -> (x+y=→"del_ETA":timestamp)
            n63 = for {
              N: w161 -> [_]
              tunnel: w136 -> [w196]
              shift-right: [w194] -> w134
              shift-left: w165 -> [w197]
              tunnel: w143 -> [w192]
              shift-right: [w191] -> w164
              shift-left: w162 -> [w193]
              tunnel: w160 -> [w190]
              i -> [w195]
              n64 = for {
                N: w190 -> [_]
                tunnel: w196 -> [w204]
                tunnel: w195 -> [w201]
                shift-right: [w203] -> w194
                shift-left: w197 -> [w205]
                tunnel: w192 -> [w199]
                shift-right: [w198] -> w191
                shift-left: w193 -> [w202]
                i -> [w200]
                n65 = in-place {
                  in-place-border: w199 -> [w211]
                  n66 = in-place-array #1(w205, w204, w201, w200) -> (w212:dbl)
                  n67 = in-place-array #2(w202, w201, w200) -> (w209:dbl)
                  n68 = Multiply(x=w212, y=w211) -> (x*y=w210:dbl)
                  n69 = Increment(x=w211) -> (x+1=w207:i32)
                  n70 = Add(x=w210, y=w209) -> (x+y=w208:dbl)
                  n71 = Divide(x=w208, y=w207) -> (x/y=w206:dbl)
                  n72 = in-place-array #1(w206) -> (w203:dbl[][][])  [unwired: 3 out]
                  n73 = in-place-array #2(w206) -> (w198:dbl[][])  [unwired: 2 out]
                }
              }
            }
            n74 = call-poly <vilib>:"Write Delimited Spreadsheet.vi"("file path (dialog if empty)"=w139, "2D data"=w164) -> ()  [unwired: 12 in, 2 out]
            n75 = property on="mainimg" class="IntGraph (strict)"() -> ("CrsrLis"=w135:T4)  [unwired: 2 in, 2 out]
            n76 = call "processData.vi"("Cursor List"=w135, "data in"=w134) -> ("Intensity Chart"=w133:dbl[])  [unwired: 1 in, 2 out]
            n77 = Increment(x=w136) -> (x+1=w137:i32)
            n78 = Bundle("delay pointss [fs]"=w132, "Intensity Chart"=w133) -> (w131:T5)  [unwired: 1 in]
            n79 = flat-sequence {
              tunnel: w131 -> [w183]
              tunnel: [w183] -> w138
              tunnel: w137 -> [w182]
              frame #0 {
                "delscan_progress" <- w182
              }
            }
            n80 = Or(x="delscan_finishIteration", y="delscan_abort") -> (x .or. y?=w156:bool)
            "delscan_pos" <- w159
            "scangraph" <- w138
          }
          n81 = Increment(x=w120) -> (x+1=w119:i32)
          "iteration" <- w119
          n82 = local read "exposure [ms]"() -> (w103:u32)
          n83 = local read "delscan_iters"() -> (w113:u32)
          n84 = local read "ROI Bottom"() -> (w106:i32)
          n85 = property on="Mode" class="Enum (strict)"() -> ("RingText.Text"=w92:string)  [unwired: 2 in, 2 out]
          n86 = property on="VoltageRange" class="Enum (strict)"() -> ("RingText.Text"=w93:string)  [unwired: 2 in, 2 out]
          n87 = local read "cam_dark?"() -> (w90:bool)
          n88 = local read "phoib_I_1"() -> (w94:dbl)
          n89 = local read "phoib_I_2"() -> (w95:dbl)
          n90 = local read "phoib_I_3"() -> (w96:dbl)
          n91 = local read "phoib_I_4"() -> (w97:dbl)
          n92 = local read "phoib_I_5"() -> (w98:dbl)
          n93 = local read "phoib_I_6"() -> (w99:dbl)
          n94 = local read "phoib_I_7"() -> (w100:dbl)
          n95 = local read "phoib_I_8"() -> (w101:dbl)
          n96 = local read "phoib_I_9"() -> (w102:dbl)
          n97 = local read "ROI Right"() -> (w108:i32)
          n98 = local read "averages"() -> (w112:i32)
          n99 = local read "ROI Top"() -> (w107:i32)
          n100 = local read "ROI Left"() -> (w109:i32)
          n101 = local read "binning"() -> (w105:u16)
          n102 = local read "ESP_t0"() -> (w114:dbl)
          n103 = local read "gain"() -> (w89:bool)
          n104 = Boolean To (0,1)(Boolean=w89) -> (0, 1=w104:i16)
          n105 = Boolean To (0,1)(Boolean=w90) -> (0, 1=w110:i16)
          n106 = Format Into String(format string="ScanType:%s\\nAverages:%u\\nRepetitions:%u\\nTimeZero:%f\\nLensMode:%s\\nVoltageRange:%s\\nKineticEnergy:%f\\nPassEnergy:%f\\nCoilCurrent:%f\\nWorkFunction:%f\\nDetectorVoltage:%f\\nScreenVoltage:%f\\nConversionVoltage:%f\\nFocusDisplacement1:%f\\nFocusDisplacement2:%f\\nExposure:%u\\nGain:%u\\nBinning:%u\\nROIbottom:%u\\nROItop:%u\\nROIright:%u\\nROIleft:%u\\nDarkImg:%u\\nStartTime:%<%Y.%m.%d %H:%M:%S>T", initial string=w88, "delay" ("input 1"), w112, w113, w114, w92, w93, w94, w95, w96, w97, w98, w99, w100, w101, w102, w103, w104, w105, w106, w107, w108, w109, w110, w86) -> ()  [unwired: 1 in, 2 out]
          n107 = Less Or Equal?(x="delscan_iters", y=w119) -> (x <= y?=w117:bool)
          n108 = Or(x=w118, y=w117) -> (x .or. y?=w116:bool)
        }
        n109 = Build Path(base path=w70, name or relative path="scanvector.txt") -> (appended path=w67:path)
        n110 = call-poly <vilib>:"Write Delimited Spreadsheet.vi"("file path (dialog if empty)"=w67, "format (%.3f)"="%.6f", "1D data"=w62, "transpose? (no:F)"=TRUE ("transpose? (F)")) -> ()  [unwired: 10 in, 2 out]
        n111 = flat-sequence {
          tunnel: w66 -> [w215]
          tunnel: [w215] -> w65
          frame #0 {
            w214 = u32 1000 ("frequency (Hz)")
            n112 = call <vilib>:"Beep.vi"("use system alert? (T)"=FALSE, "duration (msec)"=w214, "frequency (Hz)"=w214) -> ()  [unwired: 9 in]
          }
        }
      }
      frame "refresh" {
        n113 = Dequeue Element(queue=w221) -> ()  [unwired: 2 in, 4 out]
        n114 = property on="mainimg" class="IntGraph (strict)"() -> ("CrsrLis"=w220:T4)  [unwired: 2 in, 2 out]
        n115 = call "processData.vi"("Cursor List"=w220, "data in"=w219) -> ("Intensity Chart"=w218:dbl[])  [unwired: 1 in, 2 out]
        n116 = Bundle("delay pointss [fs]"=w217, "Intensity Chart"=w218) -> (w216:T5)  [unwired: 1 in]
        n117 = local write "scangraph"(w216) -> ()
      }
      frame "manip" {
        n118 = Dequeue Element(queue=w252) -> (queue out=w251:refnum<queue>)  [unwired: 2 in, 3 out]
        n119 = local read "RunNumber"() -> (w260:u16)
        n120 = local read "BasePath"() -> (w261:path)
        n121 = property on="delscan_progress 2" class="Slide (strict)"("Scale.Maximum"="manip_scan_steps") -> ()  [unwired: 2 in, 2 out]
        n122 = Index Array(array="manip_scan_delta") -> (element #1=w273:dbl, element #2=w272:dbl, element #3=w271:dbl, element #4=w270:dbl, element #5=w269:dbl, element #6=w268:dbl)  [unwired: 6 in]
        n123 = Increment(x=w260) -> (x+1=w262:u16)
        n124 = Current VI's Path() -> (path=w259:path)
        n125 = Format Into String(format string="%g_%g_%g_%g_%g_%g", w273, w272, w271, w270, w269, w268) -> (resulting string=w266:string)  [unwired: 2 in, 1 out]
        n126 = property on="Mode" class="Enum (strict)"() -> ("RingText.Text"=w246:string)  [unwired: 2 in, 2 out]
        n127 = property on="VoltageRange" class="Enum (strict)"() -> ("RingText.Text"=w245:string)  [unwired: 2 in, 2 out]
        n128 = call "saverunnumber.vi"("RunNumber"=w262, "VI path"=w259) -> ()  [unwired: 10 in]
        n129 = local write "RunNumber"(w262) -> ()
        n130 = call "create_opti_path.vi"("RunNumber"=w262, "base path"=w261) -> ("Path"=w225:path)  [unwired: 2 in]
        n131 = local read "exposure [ms]"() -> (w235:u32)
        n132 = Build Path(base path=w225, name or relative path="info.txt") -> (appended path=w224:path)
        n133 = Concatenate Strings("relative:" ("string"), w266, ":wait" ("string")) -> (w275:string)
        n134 = local read "ROI Bottom"() -> (w232:i32)
        n135 = local read "cam_dark?"() -> (w249:bool)
        n136 = local read "phoib_I_1"() -> (w244:dbl)
        n137 = local read "phoib_I_2"() -> (w243:dbl)
        n138 = local read "phoib_I_3"() -> (w242:dbl)
        n139 = local read "phoib_I_4"() -> (w241:dbl)
        n140 = local read "phoib_I_5"() -> (w240:dbl)
        n141 = local read "phoib_I_6"() -> (w239:dbl)
        n142 = local read "phoib_I_7"() -> (w238:dbl)
        n143 = local read "phoib_I_8"() -> (w237:dbl)
        n144 = local read "phoib_I_9"() -> (w236:dbl)
        n145 = local read "ROI Right"() -> (w230:i32)
        n146 = local read "averages"() -> (w247:i32)
        n147 = local read "ROI Top"() -> (w231:i32)
        n148 = local read "ROI Left"() -> (w229:i32)
        n149 = local read "binning"() -> (w233:u16)
        n150 = local read "gain"() -> (w250:bool)
        n151 = Get Date/Time In Seconds() -> (seconds since 1Jan1904=w227:timestamp)
        n152 = Build Path(base path=w225, name or relative path="scanvector.txt") -> (appended path=w276:path)
        n153 = for {
          N: 1 -> [_]
          tunnel: w258 -> [w291]
          tunnel: w225 -> [w290]
          tunnel: w276 -> [w283]
          tunnel: "manip_scan_steps" -> [w282]
          tunnel: w275 -> [w281]
          tunnel: w256 -> [w280]
          tunnel: w251 -> [w279]
          tunnel: w257 -> [w278]
          tunnel: "manip_scan_delta" -> [w277]
          i -> [w285]
          n154 = Add(x=w285, y=1000) -> (x+y=w288:i32)
          n155 = Number To Decimal String(number=w288) -> (decimal integer string=w287:string)  [unwired: 1 in]
          n156 = String Subset(string=w287, offset (0)=1) -> (substring=w284:string)  [unwired: 1 in]
          n157 = for {
            N: w282 -> [_]
            tunnel: w291 -> [w314]
            tunnel: w290 -> [w311]
            tunnel: w284 -> [w305]
            tunnel: w283 -> [w307]
            tunnel: w281 -> [w302]
            tunnel: w280 -> [w301]
            tunnel: w279 -> [w300]
            tunnel: w278 -> [w299]
            tunnel: w277 -> [w297]
            i -> [w292]
            stop <- "abort" stop-if-true
            n158 = Increment(x=w292) -> (x+1=→"delscan_progress 2":i32)
            n159 = Multiply(x=w297, y=w292) -> (x*y=w296:dbl[])
            n160 = Enqueue Element(queue=w301, element=w302) -> (error out=w303:errorcluster)  [unwired: 2 in, 2 out]
            n161 = Add(x=w292, y=10000) -> (x+y=w320:i32)
            n162 = Dequeue Element(queue=w300, error in (no error)=w303) -> (error out=w298:errorcluster)  [unwired: 1 in, 3 out]
            n163 = Number To Decimal String(number=w320) -> (decimal integer string=w319:string)  [unwired: 1 in]
            n164 = String Subset(string=w319, offset (0)=1) -> (substring=w304:string)  [unwired: 1 in]
            n165 = Enqueue Element(queue=w299, element="snap", error in (no error)=w298) -> (error out=w313:errorcluster)  [unwired: 1 in, 2 out]
            n166 = Concatenate Strings("RAW\\" ("string"), w305, "_" ("string"), w304, ".tsv" ("string")) -> (w310:string)
            n167 = Dequeue Element(queue=w314, error in (no error)=w313) -> (element=w309:dbl[][])  [unwired: 1 in, 3 out]
            n168 = Build Path(base path=w311, name or relative path=w310) -> (appended path=w312:path)
            n169 = call-poly <vilib>:"Write Delimited Spreadsheet.vi"("file path (dialog if empty)"=w312, "2D data"=w309) -> ()  [unwired: 12 in, 2 out]
            n170 = call-poly <vilib>:"Write Delimited Spreadsheet.vi"("file path (dialog if empty)"=w307, "1D data"=w296, "append to file? (new file:F)"=TRUE ("append to file? (F)"), "transpose? (no:F)"=FALSE ("transpose? (F)")) -> ()  [unwired: 10 in, 2 out]
          }
        }
        n171 = Boolean To (0,1)(Boolean=w250) -> (0, 1=w234:i16)
        n172 = Boolean To (0,1)(Boolean=w249) -> (0, 1=w228:i16)
        n173 = Format Into String(format string="ScanType:%s\\nAverages:%u\\nMode:%s\\nVoltageRange:%s\\nKineticEnergy:%f\\nPassEnergy:%f\\nCoilCurrent:%f\\nWorkFunction:%f\\nDetectorVoltage:%f\\nScreenVoltage:%f\\nConversionVoltage:%f\\nFocusDisplacement1:%f\\nFocusDisplacement2:%f\\nExposure:%u\\nGain:%u\\nBinning:%u\\nROIbottom:%u\\nROItop:%u\\nROIright:%u\\nROIleft:%u\\nDarkImg:%u\\nStartTime:%<%Y.%m.%d %H:%M:%S>T", initial string=w224, "manipulator" ("input 1"), w247, w246, w245, w244, w243, w242, w241, w240, w239, w238, w237, w236, w235, w234, w233, w232, w231, w230, w229, w228, w227) -> ()  [unwired: 1 in, 2 out]
      }
      frame "single" {
        n174 = Dequeue Element(queue=w364) -> ()  [unwired: 2 in, 4 out]
        n175 = property on="Mode" class="Enum (strict)"() -> ("RingText.Text"=w349:string)  [unwired: 2 in, 2 out]
        n176 = property on="VoltageRange" class="Enum (strict)"() -> ("RingText.Text"=w348:string)  [unwired: 2 in, 2 out]
        n177 = local read "RunNumber"() -> (w355:u16)
        n178 = local read "BasePath"() -> (w356:path)
        n179 = local read "exposure [ms]"() -> (w338:u32)
        n180 = local read "ROI Bottom"() -> (w335:i32)
        n181 = local read "cam_dark?"() -> (w352:bool)
        n182 = local read "phoib_I_1"() -> (w347:dbl)
        n183 = local read "phoib_I_2"() -> (w346:dbl)
        n184 = local read "phoib_I_3"() -> (w345:dbl)
        n185 = local read "phoib_I_4"() -> (w344:dbl)
        n186 = local read "phoib_I_5"() -> (w343:dbl)
        n187 = local read "phoib_I_6"() -> (w342:dbl)
        n188 = local read "phoib_I_7"() -> (w341:dbl)
        n189 = local read "phoib_I_8"() -> (w340:dbl)
        n190 = local read "phoib_I_9"() -> (w339:dbl)
        n191 = local read "ROI Right"() -> (w333:i32)
        n192 = local read "ESP_pos"() -> (w322:dbl)
        n193 = local read "averages"() -> (w350:i32)
        n194 = local read "ROI Top"() -> (w334:i32)
        n195 = local read "ROI Left"() -> (w332:i32)
        n196 = local read "binning"() -> (w336:u16)
        n197 = local read "ESP_t0"() -> (w323:dbl)
        n198 = Increment(x=w355) -> (x+1=w357:u16)
        n199 = Current VI's Path() -> (path=w354:path)
        n200 = local read "gain"() -> (w353:bool)
        n201 = Get Date/Time In Seconds() -> (seconds since 1Jan1904=w330:timestamp)
        n202 = call "saverunnumber.vi"("RunNumber"=w357, "VI path"=w354) -> ()  [unwired: 10 in]
        n203 = local write "RunNumber"(w357) -> ()
        n204 = call "create_opti_path.vi"("RunNumber"=w357, "base path"=w356) -> ("Path"=w327:path)  [unwired: 2 in]
        n205 = Boolean To (0,1)(Boolean=w353) -> (0, 1=w337:i16)
        n206 = Boolean To (0,1)(Boolean=w352) -> (0, 1=w331:i16)
        n207 = Build Path(base path=w327, name or relative path="info.txt") -> (appended path=w325:path)
        n208 = Format Into String(format string="ScanType=%s\\nDelayPosition=%.6f\\nTimeZero=%.6f\\nAverages=%u\\nLensMode=%s\\nVoltageRange=%s\\nKineticEnergy=%f\\nPassEnergy=%f\\nCoilCurrent=%f\\nWorkFunction=%f\\nDetectorVoltage=%f\\nScreenVoltage=%f\\nConversionVoltage=%f\\nFocusDisplacement1=%f\\nFocusDisplacement2=%f\\nExposure=%u\\nGain=%u\\nBinning=%u\\nROIbottom=%u\\nROItop=%u\\nROIright=%u\\nROIleft=%u\\nDarkImg=%u\\nStartTime=%<%Y.%m.%d %H:%M:%S>T", initial string=w325, "single" ("input 1"), w322, w323, w350, w349, w348, w347, w346, w345, w344, w343, w342, w341, w340, w339, w338, w337, w336, w335, w334, w333, w332, w331, w330) -> ()  [unwired: 1 in, 2 out]
        n209 = Build Path(base path=w327, name or relative path="AVG\\000.tsv") -> (appended path=w328:path)
        n210 = Enqueue Element(queue=w365, element="snap" ("string")) -> (error out=w359:errorcluster)  [unwired: 2 in, 2 out]
        n211 = Dequeue Element(queue=w363, error in (no error)=w359) -> (element=w358:dbl[][])  [unwired: 1 in, 3 out]
        n212 = call-poly <vilib>:"Write Delimited Spreadsheet.vi"("file path (dialog if empty)"=w328, "2D data"=w358) -> ()  [unwired: 12 in, 2 out]
      }
    }
  }
  n213 = while {
    tunnel: w10 -> [w392]
    shift-right: [w386] -> _
    shift-left: _ -> [w385]
    shift-right: [w384] -> _
    shift-left: _ -> [w382]
    shift-right: [w383] -> _
    shift-left: _ -> [w381]
    shift-right: [w378] -> _
    shift-left: 0 -> [w379]
    shift-right: [w377] -> _
    shift-left: _ -> [w376]
    shift-right: [w375] -> _
    shift-left: _ -> [w374]
    tunnel: w11 -> [w373]
    shift-right: [w372] -> _
    shift-left: _ -> [w371]
    shift-right: [w369] -> _
    shift-left: _ -> [w368]
    shift-right: [w367] -> _
    shift-left: _ -> [w366]
    i -> [w370]
    stop <- w380 stop-if-true
    # "cam"
    n214 = Preview Queue Element(queue=w392, timeout in ms (-1)=w379) -> (queue out=w391:refnum<queue>, element=w390:string)  [unwired: 1 in, 2 out]
    n215 = Match Pattern(string=w390, regular expression=":") -> (before substring=w387:string, after substring=w388:string)  [unwired: 1 in, 2 out]
    n216 = case shown="\"bench\"" w387 {
      tunnel: w391 -> [w405 w437 w467 w506 w519 _ w607 w636 w700]
      tunnel: w388 -> [_ _ _ _ _ _ _ _ _]
      tunnel: [w399 w424 w463 w505 w517 w560 w604 w625 w698] -> w386
      tunnel: w385 -> [_ _ w463 w505 w517 w560 w604 w625 w698]
      tunnel: [w404 w438 w473 u64 0 ("Hout") w516 w564 w605 w631 w697] -> w384
      tunnel: [w406 w439 w474 w502 w515 w565 w606 w619 w696] -> w383
      tunnel: w382 -> [_ w441 w477 w504 w516 w567 w609 w633 w697]
      tunnel: w381 -> [_ w440 w469 _ w515 w566 w608 w632 w696]
      tunnel: [_ _ _ _ TRUE _ _ _ _] -> w380
      tunnel: [_ _ _ _ _ _ _ _ -1] -> w378
      tunnel: [w398 w425 w468 _ _ w574 _ _ _] -> w377
      tunnel: w376 -> [w398 w425 w468 _ _ w573 _ _ _]
      tunnel: [w399 w427 w470 w500 w514 w569 w598 w634 w695] -> w375
      tunnel: w374 -> [_ w427 w470 w500 w514 w569 _ w634 w695]
      tunnel: w373 -> [_ _ _ _ _ _ _ w623 _]
      tunnel: [w396 w422 w472 w499 w512 w527 w595 w628 w694] -> w372
      tunnel: w371 -> [w396 w422 w472 w499 w512 w562 w595 w628 w694]
      tunnel: w370 -> [_ _ _ _ _ w535 _ _ _]
      tunnel: [w397 w423 w471 w498 w513 w561 w594 w627 w693] -> w369
      tunnel: w368 -> [w397 w423 w471 w498 w513 w534 w594 w627 w693]
      tunnel: [w393 w419 w457 refnum<k21> refnum ("task out") w511 w520 w593 w618 w692] -> w367
      tunnel: w366 -> [_ w419 w458 w497 w511 w520 w593 w618 w692]
      frame "init" {
        w394 = 10106 items=["Default"=-1, "RSE"=10083, "NRSE"=10078, "Differential"=10106, "Pseudodifferential"=12529] ("input terminal configuration")
        w399 = u16[][] []
        n217 = flat-sequence {
          tunnel: [w408] -> w403
          tunnel: [w409] -> w402
          tunnel: [w417] -> w404
          tunnel: [w418] -> w406
          tunnel: w403 -> [w418]
          tunnel: w402 -> [w417]
          frame #0 {
            n218 = local write "cam_con?"(FALSE ("cam_con?")) -> ()
          }
          frame #1 {
            n219 = call "SCInitBoard.vi"("boardnr"="board number") -> ("Hout"=w412:u32, "error out"=w413:errorcluster)  [unwired: 1 in, 1 out]
            n220 = call "SCSetupCamera.vi"("Handle"=w412, "error in (no error)"=w413) -> ("Hout"=w414:u64, "error out"=w415:errorcluster)  [unwired: 1 out]
            n221 = call "SCStopCOC.vi"("error in (no error)"=w415, "Stop mode"=0, "Handle"=w414) -> ("error out"=w408:errorcluster, "Hout"=w409:u64)
          }
          frame #2 {
            n222 = local write "cam_con?"(TRUE ("cam_con?")) -> ()
          }
        }
        n223 = Dequeue Element(queue=w405) -> (queue out=w401:refnum<queue>)  [unwired: 2 in, 3 out]
        n224 = Enqueue Element At Opposite End(queue=w401, element="set") -> ()  [unwired: 2 in, 3 out]
        n225 = call-poly <vilib>:"DAQmx Create Virtual Channel.vi"("input terminal configuration"=w394, "physical channels"=tag "Dev2/ai0") -> ("task out"=w393:refnum<k21>)  [unwired: 12 in, 1 out]
      }
      frame "set" {
        n226 = Dequeue Element(queue=w437) -> ()  [unwired: 2 in, 4 out]
        n227 = call "SCStopCOC.vi"("error in (no error)"=w440, "Stop mode"=0, "Handle"=w441) -> ("error out"=w456:errorcluster, "Hout"=w455:u64)
        n228 = Bundle By Name(cluster=cluster{"Delay":dbl, "Exposure ":dbl} {"Delay"=0.0, "Exposure "=0.0} ("Delay and exposure"), "Exposure"="exposure [ms]") -> (w434:cluster{"Delay":dbl, "Exposure ":dbl})
        n229 = Bundle By Name(cluster=T6 {"Camera type"=0, "Operating mode\nHP & QE / HS & DiCam Pro "=0, "Frame trigger \n(High Performance and QE only)"=0, "Sequence trigger"=0, "Low Light\n(QE only)"=FALSE, "Gain"=FALSE, "Horzontal\nbinning"=0, "Vertical\nbinning "=0, "ROI Left"=1, "ROI Right"=20, "ROI Top"=1, "ROI Bottom"=15} ("Camera controls"), "Operating mode\nHP & QE / HS & DiCam Pro"="Operating mode\nHP & QE / HS & DiCam Pro", "Horzontal\nbinning"="binning", "Vertical\nbinning"="binning", "ROI Left"="ROI Left", "ROI Right"="ROI Right", "ROI Top"="ROI Top", "ROI Bottom"="ROI Bottom", "Gain"="gain", "Frame trigger \n(High Performance and QE only)"="Frame trigger \n(High Performance and QE only)") -> (w451:T6)
        n230 = call "New delay and exposure forma.vi"("Operating mode\nHP & QE / HS & DiCam Pro"="Operating mode\nHP & QE / HS & DiCam Pro", "Delay and exposure"=w434) -> ("Output table"=w452:string)  [unwired: 3 in]
        n231 = call "SCSetCoC.vi"("error in (no error)"=w456, "Delay and exposure table"=w452, "Camera controls"=w451, "Handle"=w455) -> ("error out"=w444:errorcluster, "Hout"=w443:u64)  [unwired: 1 out]
        n232 = call "SCGetImageSize.vi"("Handle"=w443, "error in (no error)"=w444) -> ("Hout"=w442:u64, "error out"=w426:errorcluster, "Horizontal size"=w431:i32, "Vertical size"=w430:i32)  [unwired: 2 out]
        n233 = Greater?(x=w431, y=w430) -> (0:w432:bool)
        n234 = Initialize Array(u16 0 ("dimension size"), w430, w431) -> (w424:u16[][])
        n235 = call "SCRun.vi"("error in (no error)"=w426, "Run mode"=0, "Handle"=w442) -> ("error out"=w439:errorcluster, "Hout"=w438:u64)  [unwired: 1 out]
        n236 = Select(t=w431, s=w432, f=w430) -> (s? t:f=w429:i32)
        n237 = property on="mainimg" class="IntGraph (strict)"("XScale.Maximum"=w429, "YScale.Maximum"=w429) -> ()  [unwired: 2 in, 2 out]
      }
      frame "bench" {
        n238 = Dequeue Element(queue=w467) -> ()  [unwired: 2 in, 4 out]
        n239 = call "SCStopCOC.vi"("error in (no error)"=w469, "Stop mode"=0, "Handle"=w477) -> ("error out"=w461:errorcluster, "Hout"=w462:u64)
        n240 = while {
          tunnel: w463 -> [w492]
          tunnel: w462 -> [w491]
          tunnel: w461 -> [w482]
          shift-right: [w488] -> _
          shift-left: _ -> [w487]
          tunnel: [w484] -> w460
          tunnel: [w483] -> w459
          tunnel: w458 -> [w479]
          tunnel: [w478] -> w457
          stop <- "stop" stop-if-true
          n241 = call "wait4trig.vi"("error in"=w482, "task/channels in"=w479) -> ("error out"=w481:errorcluster, "voltage out"=→"voltage out":dbl, "task out"=w478:refnum<k21>)  [unwired: 7 in]
          n242 = call "SCRun.vi"("error in (no error)"=w481, "Run mode"=4, "Handle"=w491) -> ("error out"=w493:errorcluster, "Hout"=w494:u64)  [unwired: 1 out]
          n243 = call <vilib>:"High Resolution Relative Seconds.vi"() -> ("relative seconds"=w488:dbl)
          n244 = call "grabimg.vi"("array in"=w492, "error in"=w493, "Hin"=w494) -> ("error out"=w483:errorcluster, "imgdata"=→"sideimg 2":i32[][], "Hout"=w484:u64)  [unwired: 6 in]
          n245 = Subtract(x=w488, y=w487) -> (x-y=w485:dbl)
          "x/y" <- w485
          n246 = Reciprocal(x=w485) -> (1/x=→"1/x":dbl)
        }
        n247 = call "SCStopCOC.vi"("error in (no error)"=w459, "Stop mode"=0, "Handle"=w460) -> ("error out"=w464:errorcluster, "Hout"=w465:u64)
        n248 = call "SCRun.vi"("error in (no error)"=w464, "Run mode"=0, "Handle"=w465) -> ("error out"=w474:errorcluster, "Hout"=w473:u64)  [unwired: 1 out]
      }
      frame "release" {
        n249 = Dequeue Element(queue=w506) -> ()  [unwired: 2 in, 4 out]
        n250 = flat-sequence {
          tunnel: w504 -> [w508]
          tunnel: [w507] -> w501
          tunnel: [w510] -> w502
          tunnel: w501 -> [w510]
          frame #0 {
            n251 = call "SCCloseBoard.vi"("Handle"=w508) -> ("error out"=w507:errorcluster)  [unwired: 1 in, 2 out]
          }
          frame #1 {
            n252 = local write "cam_con?"(FALSE ("cam_con?")) -> ()
          }
        }
        n253 = call <vilib>:"DAQmx Clear Task.vi"("task in"=w497) -> ()  [unwired: 14 in, 1 out]
      }
      frame "close" {
        n254 = Release Queue(queue=w519) -> ()  [unwired: 2 in, 3 out]
      }
      frame "idle", Default {
        n255 = call "grabimg.vi"("array in"=w560, "error in"=w566, "Hin"=w567) -> ("error out"=w565:errorcluster, "imgdata"=w563:i32[][], "Hout"=w564:u64)  [unwired: 6 in]
        n256 = local read "lower threshold"() -> (w558:i32)
        n257 = case shown="False" "cam_dark?" {
          tunnel: w569 -> [_ w592]
          tunnel: [w589 w591] -> w559
          tunnel: w563 -> [w589 w590]
          frame False {
          }
          frame True {
            n258 = Subtract(x=w590, y=w592) -> (x-y=w591:dbl[][])
          }
        }
        n259 = call "filtr_b.vi"("threshold"=w558, "input array"=w559) -> ("output array"=w550:dbl[][])  [unwired: 9 in]
        n260 = call <vilib>:"High Resolution Relative Seconds.vi"() -> ("relative seconds"=w574:dbl)
        n261 = Subtract(x=w574, y=w573) -> (x-y=w572:dbl)
        n262 = Array Size(array=w550) -> (size(s)=w549:i32[])
        n263 = Reciprocal(x=w572) -> (1/x=→"cam_fps":dbl)
        n264 = Index Array(array=w549) -> (element #1=w544:i32, element #2=w543:i32)  [unwired: 2 in]
        n265 = Subtract(x=w535, y=w534) -> (x-y=w533:i32)
        n266 = Less Or Equal?(x="pics2avg", y=w533) -> (x <= y?=w556:bool)
        n267 = And(x="reset every n pics", y=w556) -> (x .and. y?=w554:bool)
        n268 = Not(x=w554) -> (.not. x?=w553:bool)
        n269 = call-poly <vilib>:"Ramp Pattern.vi"("start"=0.0, "end"=w544, "samples"=w544) -> ("Ramp Pattern"=w539:dbl[])  [unwired: 7 in, 1 out]
        n270 = call-poly <vilib>:"Ramp Pattern.vi"("start"=0.0, "end"=w543, "samples"=w543) -> ("Ramp Pattern"=w540:dbl[])  [unwired: 7 in, 1 out]
        n271 = property on="mainimg" class="IntGraph (strict)"() -> ("CrsrLis"=w532:T4)  [unwired: 2 in, 2 out]
        n272 = And(x="cam_liveavg", y=w553) -> (x .and. y?=w551:bool)
        n273 = case shown="False" w551 {
          tunnel: w550 -> [w579 w585]
          tunnel: [w579 w582] -> w527
          tunnel: w562 -> [_ w587]
          tunnel: w535 -> [w580 _]
          tunnel: [w580 w588] -> w561
          tunnel: w534 -> [_ w588]
          tunnel: w533 -> [_ w581]
          frame False {
          }
          frame True {
            n274 = Multiply(x=w587, y=w581) -> (x*y=w586:dbl[][])
            n275 = Increment(x=w581) -> (x+1=w583:i32)
            n276 = Add(x=w586, y=w585) -> (x+y=w584:dbl[][])
            n277 = Divide(x=w584, y=w583) -> (x/y=w582:dbl[][])
          }
        }
        "mainimg" <- w527
        n278 = Index Array(array=w532) -> (element #1=w530:T7, element #2=w531:T7)  [unwired: 2 in]
        n279 = Unbundle By Name(w530) -> ("Position.X"=w524:dbl, "Position.Y"=w526:dbl)
        n280 = Unbundle By Name(w531) -> ("Position.X"=w528:dbl, "Position.Y"=w529:dbl)
        n281 = Array Max & Min(array=w527) -> (max value=→"max":dbl)  [unwired: 3 out]
        n282 = Subtract(x=w529, y=w526) -> (x-y=w525:dbl)
        n283 = Subtract(x=w528, y=w524) -> (x-y=w523:dbl)
        n284 = Array Subset(array=w527, index (row)=w526, length (row)=w525) -> (w538:dbl[][])  [unwired: 2 in]
        n285 = Array Subset(array=w527, index (col)=w524, length (col)=w523) -> (w536:dbl[][])  [unwired: 2 in]
        n286 = Array Subset(array=w527, index (row)=w526, length (row)=w525, index (col)=w524, length (col)=w523) -> (w522:dbl[][])
        n287 = Transpose 2D Array(2D array=w538) -> (transposed array=w537:dbl[][])
        n288 = Add Array Elements(numeric array=w522) -> (sum=→"sum" →"Waveform Chart":dbl)
        n289 = for {
          tunnel: w536 -> [w576] mode=indexing
          tunnel: [w575] -> w546 mode=indexing
          n290 = Add Array Elements(numeric array=w576) -> (sum=w575:dbl)
        }
        n291 = for {
          tunnel: w537 -> [w578] mode=indexing
          tunnel: [w577] -> w545 mode=indexing
          n292 = Add Array Elements(numeric array=w578) -> (sum=w577:dbl)
        }
        n293 = Bundle("Ramp Pattern"=w540, w545) -> (→"G2 X":cluster{"Ramp Pattern":dbl[], dbl[]})  [unwired: 1 in]
        n294 = Bundle(w546, "Ramp Pattern"=w539) -> (→"G2 Y":cluster{dbl[], "Ramp Pattern":dbl[]})  [unwired: 1 in]
      }
      frame "dark" {
        n295 = Dequeue Element(queue=w607) -> ()  [unwired: 2 in, 4 out]
        n296 = Array Size(array=w604) -> (size(s)=w603:i32[])
        n297 = Index Array(array=w603) -> (element #1=w602:i32, element #2=w601:i32)  [unwired: 2 in]
        n298 = Initialize Array(0.0 ("element"), w602, w601) -> (w599:dbl[][])
        n299 = for {
          N: "dark avg" -> [_]
          tunnel: w609 -> [w617]
          tunnel: w608 -> [w616]
          tunnel: [w615] -> w606
          tunnel: w604 -> [w614]
          tunnel: [w613] -> w605
          shift-right: [w610] -> w597
          shift-left: w599 -> [w611]
          n300 = call "grabimg.vi"("array in"=w614, "error in"=w616, "Hin"=w617) -> ("error out"=w615:errorcluster, "imgdata"=w612:i32[][], "Hout"=w613:u64)  [unwired: 6 in]
          n301 = Add(x=w612, y=w611) -> (x+y=w610:dbl[][])
        }
        n302 = Divide(x=w597, y="dark avg") -> (x/y=w598:dbl[][])
      }
      frame "snap" {
        n303 = Dequeue Element(queue=w636) -> ()  [unwired: 2 in, 4 out]
        n304 = local read "cam_dark?"() -> (w635:bool)
        n305 = local read "averages"() -> (w630:i32)
        n306 = To Double Precision Float(number=w625) -> (double precision float=w624:dbl[][])
        n307 = Equal To 0?(x="aq.mode") -> (x = 0?=w621:bool)
        n308 = Get Date/Time In Seconds() -> (seconds since 1Jan1904=w626:timestamp)
        n309 = for {
          N: w630 -> [w644]
          shift-right: [w664] -> w631
          shift-left: w633 -> [w666]
          shift-right: [w651] -> w629
          shift-left: w632 -> [w665]
          tunnel: w635 -> [w662]
          tunnel: w634 -> [w661]
          tunnel: w625 -> [w660]
          tunnel: w626 -> [w656]
          tunnel: w621 -> [w646]
          shift-right: [w645] -> w620
          shift-left: w624 -> [w647]
          i -> [w641]
          stop <- "abort acq." stop-if-true
          n310 = call "grabimg.vi"("array in"=w660, "error in"=w665, "Hin"=w666) -> ("error out"=w651:errorcluster, "imgdata"=w663:i32[][], "Hout"=w664:u64)  [unwired: 6 in]
          n311 = local read "lower threshold"() -> (w639:i32)
          n312 = Increment(x=w641) -> (x+1=w642:i32)
          "acq. imgs" <- w642
          n313 = Get Date/Time In Seconds() -> (seconds since 1Jan1904=w659:timestamp)
          n314 = case shown="True" w662 {
            tunnel: w663 -> [w688 w691]
            tunnel: w661 -> [_ w690]
            tunnel: [w688 w689] -> w638
            frame False {
            }
            frame True {
              n315 = Subtract(x=w691, y=w690) -> (x-y=w689:dbl[][])
            }
          }
          n316 = Divide(x=w642, y=w644) -> (x/y=→"snap_prog":dbl)
          n317 = Subtract(x=w659, y=w656) -> (x-y=w658:dbl)
          n318 = call "filtr_b.vi"("threshold"=w639, "input array"=w638) -> ("output array"=w637:dbl[][])  [unwired: 9 in]
          n319 = Divide(x=w658, y=w641) -> (x/y=w654:dbl)
          n320 = Multiply(x=w654, y=w644) -> (x*y=w657:dbl)
          n321 = Reciprocal(x=w654) -> (1/x=w653:dbl)
          n322 = case shown="True" "count?" {
            tunnel: w637 -> [w677 w679]
            tunnel: "e-size" -> [_ w681]
            tunnel: w639 -> [_ w680]
            tunnel: [w677 w678] -> w648
            frame False {
            }
            frame True {
              n323 = Array Size(array=w679) -> (size(s)=w683:i32[])
              n324 = call "findr.vi"("thresh"=w680, "esize"=w681, "inp array"=w679) -> ("locs"=w682:i32[][])  [unwired: 8 in]
              n325 = Index Array(array=w683) -> (element #1=w685:i32, element #2=w684:i32)  [unwired: 2 in]
              n326 = call "drawe.vi"("Ysize"=w685, "Xsize"=w684, "pos array"=w682) -> ("img out"=w678:i32[][])  [unwired: 8 in]
            }
          }
          n327 = Add(x=w657, y=w656) -> (x+y=→"ETA":timestamp)
          n328 = local write "cam_fps"(w653) -> ()
          n329 = case shown="True" w646 {
            tunnel: w648 -> [w667 w675]
            tunnel: w641 -> [_ w674]
            tunnel: w647 -> [w669 w673]
            tunnel: [w668 w670] -> w645
            frame False {
              n330 = Add(x=w667, y=w669) -> (x+y=w668:dbl[][])
            }
            frame True {
              n331 = Multiply(x=w673, y=w674) -> (x*y=w676:dbl[][])
              n332 = Increment(x=w674) -> (x+1=w671:i32)
              n333 = Add(x=w675, y=w676) -> (x+y=w672:dbl[][])
              n334 = Divide(x=w672, y=w671) -> (x/y=w670:dbl[][])
            }
          }
          n335 = local write "mainimg"(w637) -> ()
          n336 = Transpose 2D Array(2D array=w637) -> (transposed array=w652:dbl[][])
          n337 = for {
            tunnel: w652 -> [w687] mode=indexing
            tunnel: [w686] -> _ mode=indexing
            n338 = Add Array Elements(numeric array=w687) -> (sum=w686:dbl)
          }
          n339 = local write "sideimg"(w645) -> ()
        }
        n340 = Enqueue Element(queue=w623, element=w620, error in (no error)=w629) -> (error out=w619:errorcluster)  [unwired: 1 in, 2 out]
      }
      frame "suspend" {
        n341 = Dequeue Element(queue=w700) -> ()  [unwired: 2 in, 4 out]
      }
    }
    "cam_error" <- w383
  }
  n342 = while {
    tunnel: w10 -> [w706]
    tunnel: w13 -> [w705]
    tunnel: w3 -> [w704]
    tunnel: w24 -> [w703]
    tunnel: w2 -> [w701]
    tunnel: w11 -> [w702]
    stop <- w707 stop-if-true
    n343 = event shown="[25] \"dev_bench\": Value Change" {
      selector: _ -> [_ _ _ _ _ _ _ _ _ _ _ _ _ _ _ _ _ _ _ _ _ _ _ _ _ _]
      dyn-events: _ -> [_ _ _ _ _ _ _ _ _ _ _ _ _ _ _ _ _ _ _ _ _ _ _ _ _ _]
      timeout: _ -> [_ _ _ _ _ _ _ _ _ _ _ _ _ _ _ _ _ _ _ _ _ _ _ _ _ _]
      tunnel: [_ TRUE _ _ _ _ _ _ _ _ _ _ _ _ _ _ _ _ _ _ _ _ _ _ _ _] -> w707
      tunnel: w706 -> [_ w720 w723 _ _ _ _ _ w749 w751 _ _ _ _ _ _ _ _ _ _ _ _ _ _ _ w856]
      tunnel: w705 -> [_ w719 _ w727 _ _ _ _ _ _ _ _ _ _ _ _ w782 _ w794 _ _ _ _ _ _ _]
      tunnel: w704 -> [_ w718 _ _ w733 _ _ _ _ _ _ _ _ w770 _ w774 _ _ _ _ _ _ _ _ _ _]
      tunnel: w703 -> [_ w717 _ _ _ w739 w745 w746 _ _ _ _ _ _ _ _ _ _ _ _ _ _ _ _ _ _]
      tunnel: w702 -> [_ w711 _ _ _ _ _ _ _ _ _ _ _ _ _ _ _ _ _ _ _ _ _ _ _ _]
      tunnel: w701 -> [_ w710 _ _ _ _ _ _ _ _ w753 w755 _ _ w772 _ _ _ _ _ _ _ _ _ w855 _]
      event Timeout {
        n344 = event-data() -> ()  [unwired: 1 in, 1 out]
        n345 = call-poly <vilib>:"Read Delimited Spreadsheet.vi"() -> ("all rows"=w708:string[][])  [unwired: 10 in, 5 out]
        n346 = local write "delay table [fs]"(w708) -> ()
      }
      event "main_close": Value Change {
        w709 = "close" ("element")
        w716 = "release" ("element")
        n347 = event-data() -> ()  [unwired: 1 in, 1 out]
        n348 = Release Queue(queue=w711) -> ()  [unwired: 2 in, 3 out]
        n349 = Enqueue Element(queue=w720, element=w716) -> (queue out=w715:refnum<queue>)  [unwired: 2 in, 2 out]
        n350 = Enqueue Element(queue=w719, element=w716) -> (queue out=w714:refnum<queue>)  [unwired: 2 in, 2 out]
        n351 = Enqueue Element(queue=w718, element=w716) -> (queue out=w713:refnum<queue>)  [unwired: 2 in, 2 out]
        n352 = Enqueue Element(queue=w717, element=w716) -> (queue out=w712:refnum<queue>)  [unwired: 2 in, 2 out]
        n353 = Enqueue Element(queue=w715, element=w709) -> ()  [unwired: 2 in, 3 out]
        n354 = Enqueue Element(queue=w714, element=w709) -> ()  [unwired: 2 in, 3 out]
        n355 = Enqueue Element(queue=w713, element=w709) -> ()  [unwired: 2 in, 3 out]
        n356 = Enqueue Element(queue=w712, element=w709) -> ()  [unwired: 2 in, 3 out]
        n357 = Enqueue Element(queue=w710, element=w709) -> ()  [unwired: 2 in, 3 out]
      }
      event "cam_release", "cam_init": Value Change {
        n358 = event-data() -> ()  [unwired: 1 in, 2 out]
        n359 = Select(t="init" ("name (unnamed)"), s="cam_init", f="release" ("name (unnamed)")) -> (s? t:f=w722:string)
        n360 = Enqueue Element(queue=w723, element=w722) -> ()  [unwired: 2 in, 3 out]
      }
      event "ESP_release", "ESP_init": Value Change {
        n361 = event-data() -> ()  [unwired: 1 in, 2 out]
        n362 = Select(t="init" ("name (unnamed)"), s="ESP_init", f="release" ("name (unnamed)")) -> (s? t:f=w731:string)
        n363 = Enqueue Element(queue=w727, element=w731) -> ()  [unwired: 2 in, 3 out]
      }
      event "manip_init", "manip_release": Value Change {
        n364 = event-data() -> ()  [unwired: 1 in, 2 out]
        n365 = Flush Queue(queue=w733) -> (queue out=w732:refnum<queue>)  [unwired: 1 in, 2 out]
        n366 = Select(t="init" ("name (unnamed)"), s="manip_init", f="release" ("name (unnamed)")) -> (s? t:f=w735:string)
        n367 = Enqueue Element(queue=w732, element=w735) -> ()  [unwired: 2 in, 3 out]
      }
      event "phoib_release", "phoib_init": Value Change {
        n368 = event-data() -> ()  [unwired: 1 in, 2 out]
        n369 = Flush Queue(queue=w739) -> (queue out=w738:refnum<queue>)  [unwired: 1 in, 2 out]
        n370 = Select(t="init" ("name (unnamed)"), s="phoib_init", f="release" ("name (unnamed)")) -> (s? t:f=w741:string)
        n371 = Enqueue Element(queue=w738, element=w741) -> ()  [unwired: 2 in, 3 out]
      }
      event "phoib_standby": Value Change {
        n372 = event-data() -> ()  [unwired: 1 in, 2 out]
        n373 = Enqueue Element(queue=w745, element="standby") -> ()  [unwired: 2 in, 3 out]
      }
      event "phoib_set": Value Change {
        n374 = event-data() -> ()  [unwired: 1 in, 2 out]
        n375 = Enqueue Element(queue=w746, element="set") -> ()  [unwired: 2 in, 3 out]
      }
      event "cam_dark": Value Change {
        n376 = event-data() -> ()  [unwired: 1 in, 2 out]
        n377 = Enqueue Element(queue=w749, element="dark") -> ()  [unwired: 2 in, 3 out]
      }
      event "ROI Left", "ROI Right", "ROI Top", "ROI Bottom", "exposure [ms]", "binning", "gain": Value Change {
        n378 = event-data() -> ()  [unwired: 1 in, 1 out]
        n379 = Enqueue Element(queue=w751, element="set") -> ()  [unwired: 2 in, 3 out]
      }
      event "cam_saveimg": Value Change {
        n380 = event-data() -> ()  [unwired: 1 in, 1 out]
        n381 = Enqueue Element(queue=w753, element="single") -> ()  [unwired: 2 in, 3 out]
      }
      event "delscan_go": Value Change {
        n382 = event-data() -> ()  [unwired: 1 in, 1 out]
        n383 = Enqueue Element(queue=w755, element="GO") -> ()  [unwired: 2 in, 3 out]
      }
      event "Move Abs": Value Change {
        n384 = event-data() -> ()  [unwired: 1 in, 1 out]
      }
      event "ManipRel +", "ManipRel -": Value Change {
        n385 = event-data() -> ()  [unwired: 1 in, 2 out]
        n386 = Negate(x="manip_deltas") -> (-x=w758:dbl[])
        n387 = Select(t="manip_deltas", s="ManipRel +", f=w758) -> (s? t:f=w756:dbl[])
        n388 = Index Array(array=w756) -> (element #1=w762:dbl, element #2=w763:dbl, element #3=w764:dbl, element #4=w765:dbl, element #5=w766:dbl, element #6=w767:dbl)  [unwired: 6 in]
        n389 = Format Into String(format string="%g_%g_%g_%g_%g_%g", w762, w763, w764, w765, w766, w767) -> (resulting string=w769:string)  [unwired: 2 in, 1 out]
        n390 = Concatenate Strings("relative:" ("string"), w769) -> (w760:string)
        n391 = Enqueue Element(queue=w770, element=w760) -> ()  [unwired: 2 in, 3 out]
      }
      event "Optimize": Value Change {
        n392 = event-data() -> ()  [unwired: 1 in, 6 out]
        n393 = Enqueue Element(queue=w772, element="manip") -> ()  [unwired: 2 in, 3 out]
      }
      event "stop manip": Value Change {
        n394 = event-data() -> ()  [unwired: 1 in, 1 out]
        n395 = Enqueue Element(queue=w774, element="stop") -> ()  [unwired: 2 in, 3 out]
      }
      event "ESP_go": Value Change {
        w776 = ":" ("string")
        n396 = event-data() -> ()  [unwired: 1 in, 1 out]
        n397 = local read "ESP Axis"() -> (w775:i32)
        n398 = Number To Decimal String(number=w775) -> (decimal integer string=w778:string)  [unwired: 1 in]
        n399 = Number To Fractional String(number="ESP_dest") -> (F-format string=w777:string)  [unwired: 3 in]
        n400 = Concatenate Strings("abs:" ("string"), w778, w776, w777, w776) -> (w781:string)
        n401 = Enqueue Element(queue=w782, element=w781) -> ()  [unwired: 2 in, 3 out]
      }
      event "ESP_set_t0": Value Change {
        n402 = event-data() -> ()  [unwired: 1 in, 1 out]
        n403 = Current VI's Path() -> (path=w788:path)
        n404 = Strip Path(path=w788) -> (stripped path=w784:path)  [unwired: 1 out]
        n405 = Strip Path(path=w784) -> (stripped path=w783:path)  [unwired: 1 out]
        n406 = local read "ESP_pos"() -> (w786:dbl)
        "ESP_t0" <- w786
        n407 = Number To Fractional String(number=w786) -> (F-format string=w785:string)  [unwired: 3 in]
        n408 = Build Path(base path=w783, name or relative path="t0.txt") -> (appended path=w787:path)
        n409 = Write to Text File(file (use dialog)=w787, text=w785) -> ()  [unwired: 2 in, 3 out]
      }
      event "ESP_+", "ESP_-": Value Change {
        n410 = event-data() -> ()  [unwired: 1 in, 6 out]
        n411 = Negate(x="ESP_delta") -> (-x=w797:dbl)
        n412 = Select(t="ESP_delta", s="ESP_+", f=w797) -> (s? t:f=w795:dbl)
        n413 = Number To Decimal String(number="ESP Axis") -> (decimal integer string=w792:string)  [unwired: 1 in]
        n414 = Number To Fractional String(number=w795) -> (F-format string=w790:string)  [unwired: 3 in]
        n415 = Concatenate Strings("rel:" ("string"), w792, ":" ("string"), w790) -> (w800:string)
        n416 = Enqueue Element(queue=w794, element=w800) -> ()  [unwired: 2 in, 3 out]
      }
      event "ESP_dest": Value Change {
        n417 = event-data() -> ()  [unwired: 1 in, 6 out]
        n418 = local read "ESP_dest"() -> (w804:dbl)
        n419 = local read "ESP_t0"() -> (w803:dbl)
        n420 = call "mm2time.vi"("fs?"=TRUE ("fs[1]/ps[0]"), "Offset (mm)"=w803, "distance (mm)"=w804) -> ("time in fs/ps seconds"=w801:dbl)
        n421 = local write "ESP_dest_t"(w801) -> ()
      }
      event "ESP_dest_t": Value Change {
        n422 = event-data() -> ()  [unwired: 1 in, 1 out]
        n423 = local read "ESP_t0"() -> (w807:dbl)
        n424 = call "time2mm.vi"("fs[1]/ps[0]"=TRUE, "Offset (mm)"=w807, "time"="ESP_dest_t") -> ("position (mm)"=w805:dbl)
        n425 = local write "ESP_dest"(w805) -> ()
      }
      event "load delay table": Value Change {
        n426 = event-data() -> ()  [unwired: 1 in, 6 out]
        n427 = call-poly <vilib>:"Read Delimited Spreadsheet.vi"() -> ("all rows"=w810:string[][])  [unwired: 10 in, 5 out]
        n428 = local read "binning"() -> (w817:u16)
        n429 = local write "delay table [fs]"(w810) -> ()
        n430 = local read "delscan_iters"() -> (w811:u32)
        n431 = local read "time / step"() -> (w820:dbl)
        n432 = Array Size(array=w810) -> (size(s)=w821:i32[])
        n433 = Index Array(array=dbl[] [8.79, 2.2, 0.553, 0.138], index=w817) -> (element=w815:dbl)
        n434 = Index Array(array=w821) -> (element #1=w809:i32)  [unwired: 2 in, 1 out]
        n435 = Multiply(x=w811, y=w809) -> (x*y=w814:u32)
        n436 = Multiply(x=w809, y=w815) -> (x*y=w816:dbl)
        n437 = Multiply(x=w814, y=w820) -> (x*y=w819:dbl)
        n438 = Increment(x=w814) -> (x+1=w813:u32)
        n439 = Multiply(x=w813, y=w815) -> (x*y=w812:dbl)
        n440 = local write "delaypoints"(w809) -> ()
        n441 = local write "total steps"(w814) -> ()
        n442 = local write "duration [HH:MM:SS]"(w819) -> ()
        n443 = local write "RAM [MB]"(w816) -> ()
        n444 = local write "disk [MB]"(w812) -> ()
      }
      event "delay table [fs]", "delscan_iters": Value Change {
        n445 = event-data() -> ()  [unwired: 1 in, 6 out]
        n446 = local read "binning"() -> (w830:u16)
        n447 = local read "delay table [fs]"() -> (w834:string[][])
        n448 = local read "delscan_iters"() -> (w824:u32)
        n449 = local read "time / step"() -> (w832:dbl)
        n450 = Array Size(array=w834) -> (size(s)=w833:i32[])
        n451 = Index Array(array=dbl[] [8.79, 2.2, 0.553, 0.138], index=w830) -> (element=w828:dbl)
        n452 = Index Array(array=w833) -> (element #1=w822:i32)  [unwired: 2 in, 1 out]
        n453 = Multiply(x=w824, y=w822) -> (x*y=w827:u32)
        n454 = Multiply(x=w822, y=w828) -> (x*y=w829:dbl)
        n455 = Multiply(x=w827, y=w832) -> (x*y=w831:dbl)
        n456 = Increment(x=w827) -> (x+1=w826:u32)
        n457 = Multiply(x=w826, y=w828) -> (x*y=w825:dbl)
        n458 = local write "delaypoints"(w822) -> ()
        n459 = local write "total steps"(w827) -> ()
        n460 = local write "duration [HH:MM:SS]"(w831) -> ()
        n461 = local write "RAM [MB]"(w829) -> ()
        n462 = local write "disk [MB]"(w825) -> ()
      }
      event "generate delay table": Value Change {
        n463 = event-data() -> ()  [unwired: 1 in, 1 out]
        n464 = call "getdelaypoints.vi"("delscan_stepsize"="delscan_stepsize", "delscan_end"="delscan_end", "delscan_start"="delscan_start") -> ("delaypoints"=w850:dbl[])
        n465 = Number To Fractional String(number=w850) -> (F-format string=w849:string[])  [unwired: 3 in]
        n466 = Build Array(w849) -> (w848:string[][])
        n467 = Transpose 2D Array(2D array=w848) -> (transposed array=w835:string[][])
        n468 = local write "delay table [fs]"(w835) -> ()
        n469 = local read "binning"() -> (w844:u16)
        n470 = local read "delscan_iters"() -> (w838:u32)
        n471 = local read "time / step"() -> (w846:dbl)
        n472 = Array Size(array=w835) -> (size(s)=w847:i32[])
        n473 = Index Array(array=dbl[] [8.79, 2.2, 0.553, 0.138], index=w844) -> (element=w842:dbl)
        n474 = Index Array(array=w847) -> (element #1=w836:i32)  [unwired: 2 in, 1 out]
        n475 = Multiply(x=w838, y=w836) -> (x*y=w841:u32)
        n476 = Multiply(x=w836, y=w842) -> (x*y=w843:dbl)
        n477 = Multiply(x=w841, y=w846) -> (x*y=w845:dbl)
        n478 = Increment(x=w841) -> (x+1=w840:u32)
        n479 = Multiply(x=w840, y=w842) -> (x*y=w839:dbl)
        n480 = local write "delaypoints"(w836) -> ()
        n481 = local write "total steps"(w841) -> ()
        n482 = local write "duration [HH:MM:SS]"(w845) -> ()
        n483 = local write "RAM [MB]"(w843) -> ()
        n484 = local write "disk [MB]"(w839) -> ()
      }
      event "mainimg": Cursor Release {
        n485 = event-data() -> ()  [unwired: 1 in, 1 out]
        n486 = Enqueue Element(queue=w855, element="refresh") -> ()  [unwired: 2 in, 3 out]
      }
      event "dev_bench": Value Change {
        n487 = event-data() -> ()  [unwired: 1 in, 2 out]
        n488 = Enqueue Element(queue=w856, element="bench") -> ()  [unwired: 2 in, 3 out]
      }
    }
  }
  n489 = while {
    tunnel: w13 -> [w866]
    shift-right: [w864] -> _
    shift-left: _ -> [w862]
    shift-right: [w863] -> _
    shift-left: _ -> [w861]
    shift-right: [w859] -> _
    shift-left: 0 -> [w860]
    tunnel: w2 -> [w858]
    stop <- w865 stop-if-true
    # "ESP"
    n490 = Preview Queue Element(queue=w866, timeout in ms (-1)=w860) -> (queue out=w869:refnum<queue>, element=w870:string)  [unwired: 1 in, 2 out]
    n491 = Match Pattern(string=w870, regular expression=":") -> (before substring=w868:string, after substring=w867:string)  [unwired: 1 in, 2 out]
    n492 = case shown="\"idle\", Default" w868 {
      tunnel: w869 -> [_ w881 w899 w933 w934 w941 w946]
      tunnel: w867 -> [_ w886 w906 _ _ _ _]
      tunnel: [_ _ _ _ _ TRUE _] -> w865
      tunnel: [w873 w888 w900 w931 refnum<visa-resource-name> refnum ("VISA resource name out") w938 w945] -> w864
      tunnel: [w872 w889 w898 w930 w936 w939 w944] -> w863
      tunnel: w862 -> [w877 w891 w904 w931 w937 w938 _]
      tunnel: w861 -> [w876 w890 w905 w930 _ w939 _]
      tunnel: [_ _ _ -1 _ _ _] -> w859
      tunnel: w858 -> [_ _ w897 _ _ _ _]
      frame "idle", Default {
        n493 = local read "ESP Axis"() -> (w874:i32)
        n494 = local read "ESP_t0"() -> (w880:dbl)
        n495 = call "Read Actual Position.vi"("error in (no error)"=w876, "Axis (1)"=w874, "VISA resource name"=w877) -> ("error out"=w872:errorcluster, "Position (units)"=w875:dbl, "VISA resource name out"=w873:refnum<visa-resource-name>)  [unwired: 2 in]
        "ESP_pos" <- w875
        n496 = call "mm2time.vi"("fs?"=TRUE, "Offset (mm)"=w880, "distance (mm)"=w875) -> ("time in fs/ps seconds"=→"ESP_delay":dbl)
      }
      frame "rel" {
        n497 = Match Pattern(string=w886, regular expression=":") -> (before substring=w885:string, after substring=w884:string)  [unwired: 1 in, 2 out]
        n498 = Dequeue Element(queue=w881) -> ()  [unwired: 2 in, 4 out]
        n499 = Decimal String To Number(string=w885) -> (number=w883:i32)  [unwired: 2 in, 1 out]
        n500 = Fract/Exp String To Number(string=w884) -> (number=w882:dbl)  [unwired: 3 in, 1 out]
        n501 = call "Move Relative.vi"("error in (no error)"=w890, "Position (0 units)"=w882, "Axis (1)"=w883, "VISA resource name"=w891) -> ("error out"=w889:errorcluster, "VISA resource name out"=w888:refnum<visa-resource-name>)  [unwired: 2 in]
      }
      frame "abs" {
        n502 = Dequeue Element(queue=w899) -> ()  [unwired: 2 in, 4 out]
        n503 = Match Pattern(string=w906, regular expression=":") -> (before substring=w907:string, after substring=w895:string)  [unwired: 1 in, 2 out]
        n504 = Match Pattern(string=w895, regular expression=":") -> (before substring=w894:string, after substring=w893:string)  [unwired: 1 in, 2 out]
        n505 = Decimal String To Number(string=w907) -> (number=w903:i32)  [unwired: 2 in, 1 out]
        n506 = Fract/Exp String To Number(string=w894) -> (number=w892:dbl)  [unwired: 3 in, 1 out]
        n507 = call "Move Absolute.vi"("error in (no error)"=w905, "Position (0 units)"=w892, "Axis (1)"=w903, "VISA resource name"=w904) -> ("error out"=w901:errorcluster, "VISA resource name out"=w902:refnum<visa-resource-name>)  [unwired: 2 in]
        n508 = case shown="\"wait\"" w893 {
          tunnel: w903 -> [_ w915]
          tunnel: w902 -> [w910 w920]
          tunnel: w901 -> [w909 w919]
          tunnel: [w910 w912] -> w900
          tunnel: [w909 w918] -> w898
          tunnel: w897 -> [_ w917]
          frame "", Default {
          }
          frame "wait" {
            n509 = while {
              tunnel: w915 -> [w929]
              shift-right: [w926] -> w914
              shift-left: w920 -> [w928]
              shift-right: [w925] -> w913
              shift-left: w919 -> [w927]
              stop <- w924 stop-if-true
              n510 = call "Get Axis Motion Status.vi"("error in (no error)"=w927, "Axis (1)"=w929, "VISA resource name"=w928) -> ("error out"=w925:errorcluster, "Motion Done"=w924:bool, "VISA resource name out"=w926:refnum<visa-resource-name>)  [unwired: 2 in]
            }
            n511 = flat-sequence {
              tunnel: w914 -> [w923]
              tunnel: w913 -> [w922]
              tunnel: [w923] -> w912
              tunnel: [w922] -> w911
              frame #0 {
                n512 = Wait (ms)(milliseconds to wait=u32 1000) -> ()  [unwired: 1 out]
              }
            }
            n513 = Enqueue Element(queue=w917, element="done", error in (no error)=w911) -> (error out=w918:errorcluster)  [unwired: 1 in, 2 out]
          }
        }
      }
      frame "suspend" {
        n514 = Dequeue Element(queue=w933) -> ()  [unwired: 2 in, 4 out]
      }
      frame "release" {
        n515 = Dequeue Element(queue=w934) -> ()  [unwired: 2 in, 4 out]
        n516 = call "Close.vi"("VISA resource name"=w937) -> ("error out"=w936:errorcluster)  [unwired: 10 in]
      }
      frame "close" {
        n517 = Release Queue(queue=w941) -> ()  [unwired: 2 in, 3 out]
      }
      frame "init" {
        n518 = Dequeue Element(queue=w946) -> ()  [unwired: 2 in, 4 out]
        n519 = flat-sequence {
          tunnel: [w949] -> w943
          tunnel: [w948] -> w942
          tunnel: [w953] -> w944
          tunnel: [w954] -> w945
          tunnel: w943 -> [w954]
          tunnel: w942 -> [w953]
          frame #0 {
            n520 = local write "ESP_con?"(FALSE ("ESP_con?")) -> ()
          }
          frame #1 {
            n521 = call "Initialize.vi"("VISA resource name"="ESP301 VISA", "Serial Link (RS232)"=enum16{"RS232", "USB"}."USB") -> ("VISA resource name out"=w949:refnum<visa-resource-name>, "error out"=w948:errorcluster)  [unwired: 7 in]
          }
          frame #2 {
            n522 = local write "ESP_con?"(TRUE ("ESP_con?")) -> ()
          }
        }
      }
    }
    "error out" <- w863
  }
  n523 = while {
    tunnel: w3 -> [w963]
    shift-right: [w961] -> _
    shift-left: _ -> [w959]
    shift-right: [w960] -> _
    shift-left: _ -> [w958]
    shift-right: [w956] -> _
    shift-left: 0 -> [w957]
    tunnel: w2 -> [w955]
    stop <- w962 stop-if-true
    # "manip"
    n524 = Preview Queue Element(queue=w963, timeout in ms (-1)=w957) -> (queue out=w966:refnum<queue>, element=w967:string)  [unwired: 1 in, 2 out]
    n525 = Match Pattern(string=w967, regular expression=":") -> (before substring=w965:string, after substring=w964:string)  [unwired: 1 in, 2 out]
    n526 = case shown="\"init\"" w965 {
      tunnel: w966 -> [_ w979 w1006 w1033 w1037 w1046 w1051]
      tunnel: w964 -> [_ _ w993 _ _ _ _]
      tunnel: [_ _ _ _ _ TRUE _] -> w962
      tunnel: [w973 w981 w985 w1035 refnum<k5> refnum ("gateway_connection out") w1044 w1050] -> w961
      tunnel: [w972 w980 w987 w1034 w1039 w1043 w1049] -> w960
      tunnel: w959 -> [w975 w983 w1009 w1035 w1041 w1044 _]
      tunnel: w958 -> [w974 w982 w1008 w1034 _ w1043 _]
      tunnel: [_ _ _ -1 _ _ _] -> w956
      tunnel: w955 -> [_ _ w984 _ _ _ _]
      frame "idle", Default {
        n527 = call "sp_manip_get_axis_status.vi"("error in"=w974, "gateway_connection"=w975) -> ("error out"=w972:errorcluster, "axis_out"=w971:T8, "gateway_connection out"=w973:refnum<k5>)  [unwired: 5 in, 2 out]
        n528 = for {
          tunnel: w971 -> [w978] mode=indexing
          tunnel: [w977] -> w970 mode=indexing
          tunnel: [w976] -> w969 mode=indexing
          n529 = Unbundle By Name(w978) -> ("Axis_Position"=w977:dbl, "moving"=w976:bool)
        }
        "moving?" <- w969
        n530 = local write "pos"(w970) -> ()
      }
      frame "stop" {
        n531 = Dequeue Element(queue=w979) -> ()  [unwired: 2 in, 4 out]
        n532 = call "sp_manip_abort.vi"("error in"=w982, "gateway_connection"=w983) -> ("error out"=w980:errorcluster, "gateway_connection out"=w981:refnum<k5>)  [unwired: 6 in, 2 out]
      }
      frame "relative" {
        n533 = Dequeue Element(queue=w1006) -> ()  [unwired: 2 in, 4 out]
        n534 = Match Pattern(string=w993, regular expression=":") -> (before substring=w992:string, after substring=w991:string)  [unwired: 1 in, 2 out]
        n535 = Equal?(x=w991, y="wait") -> (x = y?=w989:bool)
        n536 = call "sp_manip_get_axis_status.vi"("error in"=w1008, "gateway_connection"=w1009) -> ("error out"=w1011:errorcluster, "axis_out"=w998:T8, "gateway_connection out"=w1010:refnum<k5>)  [unwired: 5 in, 2 out]
        n537 = Scan From String(format string="%g_%g_%g_%g_%g_%g", input string=w992) -> (output 1=w1005:dbl, output 2=w1004:dbl, output 3=w1003:dbl, output 4=w1002:dbl, output 5=w1001:dbl, output 6=w1000:dbl)  [unwired: 8 in, 3 out]
        n538 = for {
          tunnel: w998 -> [w1032] mode=indexing
          tunnel: [w1031] -> w996 mode=indexing
          tunnel: [w1030] -> w997 mode=indexing
          n539 = Unbundle By Name(w1032) -> ("Axis_Name"=w1031:string, "Axis_Position"=w1030:dbl)
        }
        n540 = Build Array(w1005, w1004, w1003, w1002, w1001, w1000) -> (w999:dbl[])
        n541 = Add(x=w997, y=w999) -> (x+y=w995:dbl[])
        n542 = call "sp_manip_start_move.vi"("error in"=w1011, "target positions"=w995, "axis names"=w996, "gateway_connection"=w1010) -> ("error out"=w988:errorcluster, "gateway_connection out"=w986:refnum<k5>)  [unwired: 4 in, 2 out]
        n543 = case shown="True" w989 {
          tunnel: w988 -> [w1012 w1019]
          tunnel: [w1012 w1015] -> w987
          tunnel: w986 -> [w1013 w1020]
          tunnel: [w1013 w1018] -> w985
          tunnel: w984 -> [_ w1014]
          frame False {
          }
          frame True {
            n544 = while {
              tunnel: w1020 -> [w1024]
              tunnel: w1019 -> [w1023]
              tunnel: [w1022] -> w1018
              tunnel: [w1021] -> w1016
              stop <- w1025 continue-if-true
              n545 = call "sp_manip_get_axis_status.vi"("error in"=w1023, "gateway_connection"=w1024) -> ("error out"=w1021:errorcluster, "axis_out"=w1027:T8, "gateway_connection out"=w1022:refnum<k5>)  [unwired: 5 in, 2 out]
              n546 = for {
                tunnel: w1027 -> [w1029] mode=indexing
                tunnel: [w1028] -> w1026 mode=indexing
                n547 = Unbundle By Name(w1029) -> ("moving"=w1028:bool)
              }
              n548 = Or Array Elements(Boolean array=w1026) -> (logical OR=w1025:bool)
            }
            n549 = Enqueue Element(queue=w1014, element="done", error in (no error)=w1016) -> (error out=w1015:errorcluster)  [unwired: 1 in, 2 out]
          }
        }
      }
      frame "suspend" {
        n550 = Dequeue Element(queue=w1033) -> ()  [unwired: 2 in, 4 out]
      }
      frame "release" {
        n551 = Dequeue Element(queue=w1037) -> ()  [unwired: 2 in, 4 out]
        n552 = call "sp_manip_disconnect.vi"("gateway_connection"=w1041) -> ("error out"=w1040:errorcluster, "gateway_connection_out"=w1042:refnum<k5>)  [unwired: 7 in, 2 out]
        n553 = call "tcp_gateway_close_connection.vi"("error in"=w1040, "server_connection"=w1042) -> ("error out"=w1039:errorcluster)  [unwired: 5 in]
      }
      frame "close" {
        n554 = Release Queue(queue=w1046) -> ()  [unwired: 2 in, 3 out]
      }
      frame "init" {
        n555 = Dequeue Element(queue=w1051) -> ()  [unwired: 2 in, 4 out]
        n556 = flat-sequence {
          tunnel: [w1054] -> w1048
          tunnel: [w1053] -> w1047
          tunnel: [w1064] -> w1049
          tunnel: [w1065] -> w1050
          tunnel: w1048 -> [w1065]
          tunnel: w1047 -> [w1064]
          frame #0 {
            n557 = local write "manip_con?"(FALSE ("manip_con?")) -> ()
          }
          frame #1 {
            n558 = call "tcp_gateway_open_connection.vi"() -> ("gateway_connection"=w1057:refnum<k5>, "error out"=w1056:errorcluster)  [unwired: 5 in, 3 out]
            n559 = call "sp_manip_connect.vi"("error in"=w1056, "gateway_connection"=w1057) -> ("error out"=w1053:errorcluster, "axis_out"=w1055:T8, "gateway_connection out"=w1054:refnum<k5>)  [unwired: 5 in, 2 out]
            n560 = for {
              tunnel: w1055 -> [w1062] mode=indexing
              tunnel: [w1061] -> w1058 mode=indexing
              tunnel: [w1060] -> w1059 mode=indexing
              n561 = Unbundle By Name(w1062) -> ("Axis_Name"=w1061:string, "Axis_Position"=w1060:dbl)
            }
            "axis" <- w1058
            "pos" <- w1059
            n562 = local write "dest"(w1059) -> ()
          }
          frame #2 {
            n563 = local write "manip_con?"(TRUE ("manip_con?")) -> ()
          }
        }
      }
    }
    "error out 2" <- w960
  }
  n564 = while {
    tunnel: w24 -> [w1076]
    shift-right: [w1073] -> _
    shift-left: 0 -> [w1074]
    shift-right: [w1072] -> _
    shift-left: _ -> [w1071]
    shift-right: [w1070] -> _
    shift-left: _ -> [w1069]
    shift-right: [w1068] -> _
    shift-left: u32 0 ("pHandle") -> [w1067]
    tunnel: string[] ["Kinetic Energy", "Pass Energy", "Coil Current", "Work Function", "Detector Voltage", "Screen Voltage", "Conversion Voltage", "Focus Displacement 1", "Focus Displacement 2"] -> [w1066]
    stop <- w1075 stop-if-true
    # "phoib"
    n565 = Preview Queue Element(queue=w1076, timeout in ms (-1)=w1074) -> (queue out=w1079:refnum<queue>, element=w1080:string)  [unwired: 1 in, 2 out]
    n566 = Match Pattern(string=w1080, regular expression=":") -> (before substring=w1078:string, after substring=w1077:string)  [unwired: 1 in, 2 out]
    n567 = case shown="\"standby\"" w1078 {
      tunnel: w1079 -> [_ w1133 w1149 w1165 w1179 w1183 w1189]
      tunnel: w1077 -> [_ _ _ _ _ _ _]
      tunnel: [_ _ _ _ TRUE _ _] -> w1075
      tunnel: [_ _ _ _ _ -1 _] -> w1073
      tunnel: [w1090 w1135 w1152 w1163 w1177 w1182 w1186] -> w1072
      tunnel: w1071 -> [w1101 w1124 w1154 w1164 w1177 w1182 _]
      tunnel: [w1089 w1134 w1151 w1162 w1175 w1180 w1185] -> w1070
      tunnel: w1069 -> [w1099 w1123 w1153 _ w1175 w1180 _]
      tunnel: [w1087 w1121 w1150 w1161 w1176 w1181 w1188] -> w1068
      tunnel: w1067 -> [w1087 w1121 w1150 w1160 w1176 w1181 _]
      tunnel: w1066 -> [w1088 w1114 _ _ _ _ _]
      frame "idle", Default {
        n568 = call "SL2_AD_DLL_Phoibos_GetDeviceState.vi"("dll_path"=w1101, "pHandle_in"=w1087, "dev_type"=DEF_dev_type."devA (analyzer)", "error in"=w1099) -> ("path out"=w1086:path, "state"=→"state":T3, "error out"=w1085:errorcluster)  [unwired: 2 in]
        n569 = for {
          tunnel: w1087 -> [w1108]
          tunnel: w1088 -> [w1106] mode=indexing
          tunnel: [w1105] -> w1098 mode=indexing
          tunnel: [w1104] -> w1090
          shift-right: [w1103] -> w1089
          shift-left: w1085 -> [w1107]
          tunnel: w1086 -> [w1102]
          n570 = call "SL2_AD_DLL_Phoibos_GetVoltage.vi"("error in"=w1107, "voltage_name"=w1106, "pHandle"=w1108, "dll path in"=w1102) -> ("error out"=w1103:errorcluster, "value"=w1105:dbl, "dll path out"=w1104:path)  [unwired: 3 in]
        }
        n571 = Index Array(array=w1098) -> (element #1=→"phoib_I_1":dbl, element #2=→"phoib_I_2":dbl, element #3=→"phoib_I_3":dbl, element #4=→"phoib_I_4":dbl, element #5=→"phoib_I_5":dbl, element #6=→"phoib_I_6":dbl, element #7=→"phoib_I_7":dbl, element #8=→"phoib_I_8":dbl, element #9=→"phoib_I_9":dbl)  [unwired: 9 in]
      }
      frame "set" {
        n572 = Dequeue Element(queue=w1133) -> ()  [unwired: 2 in, 4 out]
        n573 = Multiply(x="VoltageRange", y=13) -> (x*y=w1130:i32)
        n574 = Add(x="Mode", y=w1130) -> (x+y=w1127:i32)
        n575 = Index Array(array=u32[] [251749632, 251749633, 251749634, 251749635, 251749636, 251749637, 251749638, 251749639, 251749640, 251749641, 251749642, 251749643, 251749644, 251749645, 251749646, 251749647, 251749648, 251749649, 251749650, 251749651, 251749652, 251749653, 251749654, 251749655, 251749656, 251749657, 251749658, 251749659, 251749660, 251749661, 251749662, 251749663, 251749664, 251749665, 251749666, 251749667, 251749668, 251749669, 251749670, 251749671, 251749672, 251749673, 251749674, 251749675, 251749676, 251749677, 251749678, 251749679, 251749680, 251749681, 251749682, 251749683, 251749684, 251749685, 251749686, 251749687, 251749688, 251749689, 251749690, 251749691, 251749692, 251749693, 251749694, 251749695, 251749696] ("modeIDs"), index=w1127) -> (element=w1125:u32)
        n576 = Build Array("phoib_I_1s", "phoib_I_2s", "phoib_I_3s", "phoib_I_4s", "phoib_I_5s", "phoib_I_6s", "phoib_I_7s", "phoib_I_8s", "phoib_I_9s") -> (w1113:dbl[])
        n577 = call "SL2_AD_DLL_Phoibos_SetDeviceMode.vi"("pHandle"=w1121, "error in"=w1123, "value"=w1125, "dev_type"=DEF_dev_type."devA (analyzer)", "dll path in"=w1124) -> ("error out"=w1112:errorcluster, "dll path out"=w1122:path)  [unwired: 4 in]
        n578 = for {
          tunnel: w1121 -> [w1141]
          shift-right: [w1148] -> w1135
          shift-left: w1122 -> [w1145]
          tunnel: w1114 -> [w1140] mode=indexing
          tunnel: w1113 -> [w1139] mode=indexing
          shift-right: [w1147] -> w1134
          shift-left: w1112 -> [w1143]
          n579 = call "SL2_AD_DLL_Phoibos_GetVoltageRange.vi"("error in"=w1143, "voltage_name"=w1140, "pHandle"=w1141, "dll path in"=w1145) -> ("error out"=w1142:errorcluster, "min"=w1137:dbl, "max"=w1138:dbl, "dll path out"=w1144:path)  [unwired: 2 in]
          n580 = In Range and Coerce(upper limit=w1138, x=w1139, lower limit=w1137) -> (coerced(x)=w1136:dbl)  [unwired: 1 out]
          n581 = call "SL2_AD_DLL_Phoibos_SetVoltage.vi"("commit"=TRUE, "pHandle"=w1141, "error in"=w1142, "value"=w1136, "voltageName"=w1140, "dll path in"=w1144) -> ("error out"=w1147:errorcluster, "dll path out"=w1148:path)  [unwired: 3 in]
        }
      }
      frame "standby" {
        w1155 = T3 0 items=["Off"=-1, "Standby"=0, "On"=1] ("state")
        n582 = Dequeue Element(queue=w1149) -> ()  [unwired: 2 in, 4 out]
        n583 = call "SL2_AD_DLL_Phoibos_SetDeviceState.vi"("pHandle_in"=w1150, "error in"=w1153, "state"=w1155, "dev_type"=DEF_dev_type."devA (analyzer)", "dll_path"=w1154) -> ("error out"=w1151:errorcluster, "path out"=w1152:path)  [unwired: 2 in]
      }
      frame "release" {
        n584 = Dequeue Element(queue=w1165) -> ()  [unwired: 2 in, 4 out]
        n585 = flat-sequence {
          tunnel: w1164 -> [w1166]
          tunnel: w1160 -> [w1167]
          tunnel: [w1170] -> w1159
          tunnel: [w1169] -> w1158
          tunnel: [u32 0] -> w1157
          tunnel: [w1172] -> w1161
          tunnel: [w1173] -> w1162
          tunnel: [w1174] -> w1163
          tunnel: w1159 -> [w1174]
          tunnel: w1158 -> [w1173]
          tunnel: w1157 -> [w1172]
          frame #0 {
            n586 = call "SL2_AD_DLL_Phoibos_Shutdown.vi"("pHandle"=w1167, "dll path in"=w1166) -> ("error out"=w1169:errorcluster, "dll path out"=w1170:path)  [unwired: 4 in]
          }
          frame #1 {
            n587 = local write "phoib_con?"(FALSE ("phoib_con?")) -> ()
          }
        }
      }
      frame "close" {
        n588 = Release Queue(queue=w1179) -> ()  [unwired: 2 in, 3 out]
      }
      frame "suspend" {
        n589 = Dequeue Element(queue=w1183) -> ()  [unwired: 2 in, 4 out]
      }
      frame "init" {
        n590 = Dequeue Element(queue=w1189) -> ()  [unwired: 2 in, 4 out]
        n591 = flat-sequence {
          tunnel: [w1196] -> w1187
          tunnel: [w1192] -> w1186
          tunnel: [w1191] -> w1185
          tunnel: [w1204] -> w1188
          tunnel: w1187 -> [w1204]
          frame #0 {
            n592 = local write "phoib_con?"(FALSE ("phoib_con?")) -> ()
          }
          frame #1 {
            w1195 = DEF_dev_type."devA (analyzer)" ("dev_type")
            n593 = call "GetSL2AD_VI_dllPath.vi"() -> ("error"=w1199:errorcluster, "Path"=w1200:path)  [unwired: 9 in, 1 out]
            n594 = call "SL2_AD_DLL_List_Devices.vi"("error in"=w1199, "dev_type"=w1195, "dll path in"=w1200) -> ("error out"=w1193:errorcluster, "devices"=w1202:string[], "dll path out"=w1194:path)  [unwired: 2 in]
            n595 = Index Array(array=w1202) -> (element=w1201:string)  [unwired: 1 in]
            n596 = call "SL2_AD_DLL_Phoibos_Initialize.vi"("error in"=w1193, "analyzerId"=w1201, "dll_path"=w1194) -> ("error out"=w1197:errorcluster, "pHandle"=w1196:u32, "path out"=w1198:path)  [unwired: 2 in]
            n597 = call "SL2_AD_DLL_Phoibos_ListDeviceModes.vi"("dll path in"=w1198, "dev_type"=w1195, "pHandle"=w1196, "error in"=w1197) -> ("dll path out"=w1192:path, "error out"=w1191:errorcluster)  [unwired: 1 in, 2 out]
          }
          frame #2 {
            n598 = local write "phoib_con?"(TRUE ("phoib_con?")) -> ()
          }
        }
      }
    }
    "phoib_error" <- w1070
  }
